vi "LABVIEW ECG.vi"() -> ()   [LabVIEW 2016]
uses:
  <vilib>/Instr/_visa.llb/Select Event Type.ctl
  <vilib>/Instr/_visa.llb/VISA Configure Serial Port (Instr).vi
  <vilib>/express/express analysis/Spectral/Block/exnSpectralBlock spectral measurements peak poly.vi
  <vilib>/express/express analysis/Spectral/Block/exnSpectralBlock spectral measurements peak WFM.vi
  <vilib>/express/express analysis/Spectral/Block/exnSpectralBlock spectral measurements peak DDT.vi
  <vilib>/express/express analysis/Spectral/XNode/ExpressSpectralMeasurementsBlockNode.xnode
  <vilib>/measure/NI_MABase.lvlib
  <vilib>/ptbypt/NI_PtbyPt.lvlib
panel:
  out "?":bool
  in  "?":bool
  in  "Tab Control":T1(tab)
  in  "COM Port":refnum<visa-resource-name>="COM7"
  in  "Parametres VISA":T2={"baud rate (9600)"=500000, "data bits (8)"=8, "parity (0:none)"=enum."None", "stop bits (10: 1 bit)"=10, "flow control (0:none)"=0} {"stop bits (10: 1 bit)" items=["1.0"=10, "1.5"=15, "2.0"=20]; "flow control (0:none)" items=["None", "XON/XOFF", "RTS/CTS", "XON/XOFF & RTS/CTS", "DTR/DSR", "XON/XOFF & DTR/DSR"]}
  out "Signal bruité":waveform(dbl)(graph)={"t0"=timestamp(1563.0 s since 1904-01-01), "dt"=0.001, "Y"=array[1000 elements]}
  out "Signal filtré":dynamicdata(graph)=[{"t0"=timestamp(1563.0 s since 1904-01-01), "dt"=0.001, "Y"=array[1000 elements], "attributes"=variant("NI_ChannelName"=variant(string "Filtered"))}]
  in  "Frequence Reseau":dbl=10.0 format="%0.2p"
  in  "Frequence de coupure":dbl=0.125 format="%0.3f"
  out "Table 2":string[][](table)=[["20/06/2020 23:30:40", "98,000000"], ["20/06/2020 23:30:41", "32,000000"], ["20/06/2020 23:30:41", "32,000000"], ["20/06/2020 23:30:41", "32,000000"], ["20/06/2020 23:30:41", "33,000000"], ["20/06/2020 23:30:41", "33,000000"], ["20/06/2020 23:30:41", "33,000000"], ["20/06/2020 23:30:41", "33,000000"], ["20/06/2020 23:30:41", "33,000000"], ["20/06/2020 23:30:41", "34,000000"], ["20/06/2020 23:30:41", "35,000000"], ["20/06/2020 23:30:41", "35,000000"], ["20/06/2020 23:30:41", "34,000000"], ["20/06/2020 23:30:41", "33,000000"], ["20/06/2020 23:30:41", "35,000000"], ["20/06/2020 23:30:41", "34,000000"], ["20/06/2020 23:30:41", "33,000000"], ["20/06/2020 23:30:41", "34,000000"], ["20/06/2020 23:30:41", "34,000000"], ["20/06/2020 23:30:41", "33,000000"], ["20/06/2020 23:30:41", "33,000000"], ["20/06/2020 23:30:41", "33,000000"], ["20/06/2020 23:30:41", "34,000000"], ["20/06/2020 23:30:41", "34,000000"], ["20/06/2020 23:30:41", "34,000000"], ["20/06/2020 23:30:41", "35,000000"], ["20/06/2020 23:30:41", "35,000000"], ["20/06/2020 23:30:41", "34,000000"], ["20/06/2020 23:30:41", "36,000000"], ["20/06/2020 23:30:41", "35,000000"], ["20/06/2020 23:30:41", "35,000000"], ["20/06/2020 23:30:41", "36,000000"], ["20/06/2020 23:30:41", "36,000000"], ["20/06/2020 23:30:41", "38,000000"], ["20/06/2020 23:30:41", "37,000000"], ["20/06/2020 23:30:41", "38,000000"], ["20/06/2020 23:30:41", "38,000000"], ["20/06/2020 23:30:41", "38,000000"], ["20/06/2020 23:30:41", "40,000000"], ["20/06/2020 23:30:41", "40,000000"], ["20/06/2020 23:30:41", "40,000000"], ["20/06/2020 23:30:41", "41,000000"], ["20/06/2020 23:30:41", "42,000000"], ["20/06/2020 23:30:41", "41,000000"], ["20/06/2020 23:30:41", "41,000000"], ["20/06/2020 23:30:41", "43,000000"], ["20/06/2020 23:30:41", "42,000000"], ["20/06/2020 23:30:41", "43,000000"], ["20/06/2020 23:30:41", "44,000000"], ["20/06/2020 23:30:41", "45,000000"], ["20/06/2020 23:30:41", "45,000000"], ["20/06/2020 23:30:41", "46,000000"], ["20/06/2020 23:30:41", "45,000000"], ["20/06/2020 23:30:41", "47,000000"], ["20/06/2020 23:30:41", "47,000000"], ["20/06/2020 23:30:41", "47,000000"], ["20/06/2020 23:30:41", "47,000000"], ["20/06/2020 23:30:41", "48,000000"], ["20/06/2020 23:30:41", "49,000000"], ["20/06/2020 23:30:41", "49,000000"], ["20/06/2020 23:30:41", "50,000000"], ["20/06/2020 23:30:41", "50,000000"], ["20/06/2020 23:30:41", "49,000000"], ["20/06/2020 23:30:41", "48,000000"], ["20/06/2020 23:30:41", "49,000000"], ["20/06/2020 23:30:41", "48,000000"], ["20/06/2020 23:30:41", "49,000000"], ["20/06/2020 23:30:41", "49,000000"], ["20/06/2020 23:30:41", "50,000000"], ["20/06/2020 23:30:41", "50,000000"], ["20/06/2020 23:30:41", "50,000000"], ["20/06/2020 23:30:41", "50,000000"], ["20/06/2020 23:30:41", "51,000000"], ["20/06/2020 23:30:41", "50,000000"], ["20/06/2020 23:30:41", "50,000000"], ["20/06/2020 23:30:41", "49,000000"], ["20/06/2020 23:30:41", "49,000000"], ["20/06/2020 23:30:41", "48,000000"], ["20/06/2020 23:30:41", "47,000000"], ["20/06/2020 23:30:41", "47,000000"], ["20/06/2020 23:30:41", "46,000000"], ["20/06/2020 23:30:41", "46,000000"], ["20/06/2020 23:30:41", "44,000000"], ["20/06/2020 23:30:41", "42,000000"], ["20/06/2020 23:30:41", "42,000000"], ["20/06/2020 23:30:41", "39,000000"], ["20/06/2020 23:30:41", "39,000000"], ["20/06/2020 23:30:41", "39,000000"], ["20/06/2020 23:30:41", "38,000000"], ["20/06/2020 23:30:41", "39,000000"], ["20/06/2020 23:30:41", "36,000000"], ["20/06/2020 23:30:41", "34,000000"], ["20/06/2020 23:30:41", "34,000000"], ["20/06/2020 23:30:41", "33,000000"], ["20/06/2020 23:30:41", "32,000000"], ["20/06/2020 23:30:42", "31,000000"], ["20/06/2020 23:30:42", "30,000000"], ["20/06/2020 23:30:42", "30,000000"], ["20/06/2020 23:30:42", "31,000000"], ["20/06/2020 23:30:42", "30,000000"], ["20/06/2020 23:30:42", "30,000000"], ["20/06/2020 23:30:42", "29,000000"], ["20/06/2020 23:30:42", "29,000000"], ["20/06/2020 23:30:42", "27,000000"], ["20/06/2020 23:30:42", "27,000000"], ["20/06/2020 23:30:42", "27,000000"], ["20/06/2020 23:30:42", "25,000000"], ["20/06/2020 23:30:42", "25,000000"], ["20/06/2020 23:30:42", "24,000000"], ["20/06/2020 23:30:42", "26,000000"], ["20/06/2020 23:30:42", "25,000000"], ["20/06/2020 23:30:42", "25,000000"], ["20/06/2020 23:30:42", "25,000000"], ["20/06/2020 23:30:42", "24,000000"], ["20/06/2020 23:30:42", "25,000000"], ["20/06/2020 23:30:42", "24,000000"], ["20/06/2020 23:30:42", "24,000000"], ["20/06/2020 23:30:42", "24,000000"], ["20/06/2020 23:30:42", "24,000000"], ["20/06/2020 23:30:42", "25,000000"], ["20/06/2020 23:30:42", "23,000000"], ["20/06/2020 23:30:42", "25,000000"], ["20/06/2020 23:30:42", "24,000000"], ["20/06/2020 23:30:42", "23,000000"], ["20/06/2020 23:30:42", "23,000000"], ["20/06/2020 23:30:42", "22,000000"], ["20/06/2020 23:30:42", "21,000000"], ["20/06/2020 23:30:42", "20,000000"], ["20/06/2020 23:30:42", "22,000000"], ["20/06/2020 23:30:42", "21,000000"], ["20/06/2020 23:30:42", "21,000000"], ["20/06/2020 23:30:42", "21,000000"], ["20/06/2020 23:30:42", "19,000000"], ["20/06/2020 23:30:42", "18,000000"], ["20/06/2020 23:30:42", "19,000000"], ["20/06/2020 23:30:42", "19,000000"], ["20/06/2020 23:30:42", "19,000000"], ["20/06/2020 23:30:42", "19,000000"], ["20/06/2020 23:30:42", "18,000000"], ["20/06/2020 23:30:42", "20,000000"], ["20/06/2020 23:30:42", "19,000000"], ["20/06/2020 23:30:42", "19,000000"], ["20/06/2020 23:30:42", "21,000000"], ["20/06/2020 23:30:42", "20,000000"], ["20/06/2020 23:30:42", "20,000000"], ["20/06/2020 23:30:42", "19,000000"], ["20/06/2020 23:30:42", "19,000000"], ["20/06/2020 23:30:42", "21,000000"], ["20/06/2020 23:30:42", "21,000000"], ["20/06/2020 23:30:42", "20,000000"], ["20/06/2020 23:30:42", "22,000000"], ["20/06/2020 23:30:42", "23,000000"], ["20/06/2020 23:30:42", "22,000000"], ["20/06/2020 23:30:42", "20,000000"], ["20/06/2020 23:30:42", "21,000000"], ["20/06/2020 23:30:42", "21,000000"], ["20/06/2020 23:30:42", "21,000000"], ["20/06/2020 23:30:42", "23,000000"], ["20/06/2020 23:30:42", "23,000000"], ["20/06/2020 23:30:42", "23,000000"], ["20/06/2020 23:30:42", "21,000000"], ["20/06/2020 23:30:42", "21,000000"], ["20/06/2020 23:30:42", "22,000000"], ["20/06/2020 23:30:42", "22,000000"], ["20/06/2020 23:30:42", "22,000000"], ["20/06/2020 23:30:42", "22,000000"], ["20/06/2020 23:30:42", "22,000000"], ["20/06/2020 23:30:42", "22,000000"], ["20/06/2020 23:30:42", "23,000000"], ["20/06/2020 23:30:42", "23,000000"], ["20/06/2020 23:30:42", "22,000000"], ["20/06/2020 23:30:42", "22,000000"], ["20/06/2020 23:30:42", "23,000000"], ["20/06/2020 23:30:42", "22,000000"], ["20/06/2020 23:30:42", "23,000000"], ["20/06/2020 23:30:42", "22,000000"], ["20/06/2020 23:30:42", "22,000000"], ["20/06/2020 23:30:42", "23,000000"], ["20/06/2020 23:30:42", "23,000000"], ["20/06/2020 23:30:42", "21,000000"], ["20/06/2020 23:30:42", "22,000000"], ["20/06/2020 23:30:42", "22,000000"], ["20/06/2020 23:30:42", "23,000000"], ["20/06/2020 23:30:42", "21,000000"], ["20/06/2020 23:30:42", "20,000000"], ["20/06/2020 23:30:42", "22,000000"], ["20/06/2020 23:30:42", "22,000000"], ["20/06/2020 23:30:42", "22,000000"], ["20/06/2020 23:30:42", "23,000000"], ["20/06/2020 23:30:42", "23,000000"], ["20/06/2020 23:30:42", "22,000000"], ["20/06/2020 23:30:42", "22,000000"], ["20/06/2020 23:30:42", "23,000000"], ["20/06/2020 23:30:42", "23,000000"], ["20/06/2020 23:30:42", "23,000000"], ["20/06/2020 23:30:42", "22,000000"], ["20/06/2020 23:30:42", "21,000000"], ["20/06/2020 23:30:42", "21,000000"], ["20/06/2020 23:30:42", "20,000000"], ["20/06/2020 23:30:42", "23,000000"], ["20/06/2020 23:30:42", "21,000000"], ["20/06/2020 23:30:42", "19,000000"], ["20/06/2020 23:30:42", "19,000000"], ["20/06/2020 23:30:42", "18,000000"], ["20/06/2020 23:30:42", "18,000000"], ["20/06/2020 23:30:42", "19,000000"], ["20/06/2020 23:30:42", "19,000000"], ["20/06/2020 23:30:42", "19,000000"], ["20/06/2020 23:30:42", "19,000000"], ["20/06/2020 23:30:42", "19,000000"], ["20/06/2020 23:30:42", "19,000000"], ["20/06/2020 23:30:42", "19,000000"], ["20/06/2020 23:30:42", "19,000000"], ["20/06/2020 23:30:42", "18,000000"], ["20/06/2020 23:30:42", "19,000000"], ["20/06/2020 23:30:42", "18,000000"], ["20/06/2020 23:30:42", "17,000000"], ["20/06/2020 23:30:42", "18,000000"], ["20/06/2020 23:30:42", "18,000000"], ["20/06/2020 23:30:42", "18,000000"], ["20/06/2020 23:30:42", "18,000000"], ["20/06/2020 23:30:42", "19,000000"], ["20/06/2020 23:30:42", "19,000000"], ["20/06/2020 23:30:42", "18,000000"], ["20/06/2020 23:30:42", "19,000000"], ["20/06/2020 23:30:42", "18,000000"], ["20/06/2020 23:30:42", "19,000000"], ["20/06/2020 23:30:42", "18,000000"], ["20/06/2020 23:30:42", "18,000000"], ["20/06/2020 23:30:42", "18,000000"], ["20/06/2020 23:30:42", "18,000000"], ["20/06/2020 23:30:42", "18,000000"], ["20/06/2020 23:30:42", "17,000000"], ["20/06/2020 23:30:42", "16,000000"], ["20/06/2020 23:30:42", "17,000000"], ["20/06/2020 23:30:42", "17,000000"], ["20/06/2020 23:30:42", "16,000000"], ["20/06/2020 23:30:42", "17,000000"], ["20/06/2020 23:30:42", "18,000000"], ["20/06/2020 23:30:42", "18,000000"], ["20/06/2020 23:30:42", "18,000000"], ["20/06/2020 23:30:42", "17,000000"], ["20/06/2020 23:30:42", "17,000000"], ["20/06/2020 23:30:42", "17,000000"], ["20/06/2020 23:30:42", "17,000000"], ["20/06/2020 23:30:42", "17,000000"], ["20/06/2020 23:30:42", "18,000000"], ["20/06/2020 23:30:42", "17,000000"], ["20/06/2020 23:30:42", "16,000000"], ["20/06/2020 23:30:42", "16,000000"], ["20/06/2020 23:30:42", "16,000000"], ["20/06/2020 23:30:42", "17,000000"], ["20/06/2020 23:30:42", "18,000000"], ["20/06/2020 23:30:42", "17,000000"], ["20/06/2020 23:30:42", "17,000000"], ["20/06/2020 23:30:42", "17,000000"], ["20/06/2020 23:30:42", "17,000000"], ["20/06/2020 23:30:42", "16,000000"], ["20/06/2020 23:30:42", "17,000000"], ["20/06/2020 23:30:42", "17,000000"], ["20/06/2020 23:30:42", "17,000000"], ["20/06/2020 23:30:42", "18,000000"], ["20/06/2020 23:30:42", "17,000000"], ["20/06/2020 23:30:42", "16,000000"], ["20/06/2020 23:30:42", "16,000000"], ["20/06/2020 23:30:42", "16,000000"], ["20/06/2020 23:30:42", "17,000000"], ["20/06/2020 23:30:42", "18,000000"], ["20/06/2020 23:30:42", "17,000000"], ["20/06/2020 23:30:42", "16,000000"], ["20/06/2020 23:30:42", "17,000000"], ["20/06/2020 23:30:42", "17,000000"], ["20/06/2020 23:30:42", "17,000000"], ["20/06/2020 23:30:42", "17,000000"], ["20/06/2020 23:30:42", "15,000000"], ["20/06/2020 23:30:42", "16,000000"], ["20/06/2020 23:30:42", "16,000000"], ["20/06/2020 23:30:42", "16,000000"], ["20/06/2020 23:30:42", "17,000000"], ["20/06/2020 23:30:42", "16,000000"], ["20/06/2020 23:30:42", "16,000000"], ["20/06/2020 23:30:42", "16,000000"], ["20/06/2020 23:30:42", "16,000000"], ["20/06/2020 23:30:42", "16,000000"], ["20/06/2020 23:30:42", "15,000000"], ["20/06/2020 23:30:42", "16,000000"], ["20/06/2020 23:30:42", "16,000000"], ["20/06/2020 23:30:42", "16,000000"], ["20/06/2020 23:30:42", "16,000000"], ["20/06/2020 23:30:42", "16,000000"], ["20/06/2020 23:30:42", "17,000000"], ["20/06/2020 23:30:42", "16,000000"], ["20/06/2020 23:30:42", "17,000000"], ["20/06/2020 23:30:42", "17,000000"], ["20/06/2020 23:30:42", "17,000000"], ["20/06/2020 23:30:42", "17,000000"], ["20/06/2020 23:30:42", "16,000000"], ["20/06/2020 23:30:42", "16,000000"], ["20/06/2020 23:30:42", "16,000000"], ["20/06/2020 23:30:42", "16,000000"], ["20/06/2020 23:30:42", "17,000000"], ["20/06/2020 23:30:42", "16,000000"], ["20/06/2020 23:30:42", "17,000000"], ["20/06/2020 23:30:42", "16,000000"], ["20/06/2020 23:30:42", "16,000000"], ["20/06/2020 23:30:42", "16,000000"], ["20/06/2020 23:30:42", "16,000000"], ["20/06/2020 23:30:42", "16,000000"], ["20/06/2020 23:30:42", "17,000000"], ["20/06/2020 23:30:42", "17,000000"], ["20/06/2020 23:30:42", "16,000000"], ["20/06/2020 23:30:42", "16,000000"], ["20/06/2020 23:30:42", "16,000000"], ["20/06/2020 23:30:42", "14,000000"], ["20/06/2020 23:30:42", "15,000000"], ["20/06/2020 23:30:42", "15,000000"], ["20/06/2020 23:30:42", "16,000000"], ["20/06/2020 23:30:42", "16,000000"], ["20/06/2020 23:30:42", "18,000000"], ["20/06/2020 23:30:42", "19,000000"], ["20/06/2020 23:30:42", "17,000000"], ["20/06/2020 23:30:42", "18,000000"], ["20/06/2020 23:30:42", "17,000000"], ["20/06/2020 23:30:42", "16,000000"], ["20/06/2020 23:30:42", "16,000000"], ["20/06/2020 23:30:42", "17,000000"], ["20/06/2020 23:30:42", "17,000000"], ["20/06/2020 23:30:42", "18,000000"], ["20/06/2020 23:30:42", "19,000000"], ["20/06/2020 23:30:42", "20,000000"], ["20/06/2020 23:30:42", "21,000000"], ["20/06/2020 23:30:42", "22,000000"], ["20/06/2020 23:30:42", "23,000000"], ["20/06/2020 23:30:42", "22,000000"], ["20/06/2020 23:30:42", "22,000000"], ["20/06/2020 23:30:42", "24,000000"], ["20/06/2020 23:30:42", "25,000000"], ["20/06/2020 23:30:42", "26,000000"], ["20/06/2020 23:30:42", "26,000000"], ["20/06/2020 23:30:42", "27,000000"], ["20/06/2020 23:30:42", "27,000000"], ["20/06/2020 23:30:42", "29,000000"], ["20/06/2020 23:30:42", "29,000000"], ["20/06/2020 23:30:42", "27,000000"], ["20/06/2020 23:30:42", "27,000000"], ["20/06/2020 23:30:42", "26,000000"], ["20/06/2020 23:30:42", "25,000000"], ["20/06/2020 23:30:42", "23,000000"], ["20/06/2020 23:30:42", "24,000000"], ["20/06/2020 23:30:42", "23,000000"], ["20/06/2020 23:30:42", "23,000000"], ["20/06/2020 23:30:42", "22,000000"], ["20/06/2020 23:30:42", "19,000000"], ["20/06/2020 23:30:42", "19,000000"], ["20/06/2020 23:30:42", "18,000000"], ["20/06/2020 23:30:42", "16,000000"], ["20/06/2020 23:30:42", "15,000000"], ["20/06/2020 23:30:42", "14,000000"], ["20/06/2020 23:30:42", "16,000000"], ["20/06/2020 23:30:42", "15,000000"], ["20/06/2020 23:30:42", "14,000000"], ["20/06/2020 23:30:42", "14,000000"], ["20/06/2020 23:30:42", "14,000000"], ["20/06/2020 23:30:42", "14,000000"], ["20/06/2020 23:30:42", "14,000000"], ["20/06/2020 23:30:42", "15,000000"], ["20/06/2020 23:30:42", "14,000000"], ["20/06/2020 23:30:42", "14,000000"], ["20/06/2020 23:30:42", "13,000000"], ["20/06/2020 23:30:42", "13,000000"], ["20/06/2020 23:30:42", "13,000000"], ["20/06/2020 23:30:42", "14,000000"], ["20/06/2020 23:30:42", "13,000000"], ["20/06/2020 23:30:42", "12,000000"], ["20/06/2020 23:30:42", "13,000000"], ["20/06/2020 23:30:42", "12,000000"], ["20/06/2020 23:30:42", "12,000000"], ["20/06/2020 23:30:42", "11,000000"], ["20/06/2020 23:30:42", "11,000000"], ["20/06/2020 23:30:42", "12,000000"], ["20/06/2020 23:30:42", "13,000000"], ["20/06/2020 23:30:42", "15,000000"], ["20/06/2020 23:30:42", "16,000000"], ["20/06/2020 23:30:42", "16,000000"], ["20/06/2020 23:30:42", "14,000000"], ["20/06/2020 23:30:42", "15,000000"], ["20/06/2020 23:30:42", "20,000000"], ["20/06/2020 23:30:42", "27,000000"], ["20/06/2020 23:30:42", "35,000000"], ["20/06/2020 23:30:42", "45,000000"], ["20/06/2020 23:30:42", "61,000000"], ["20/06/2020 23:30:42", "74,000000"], ["20/06/2020 23:30:42", "82,000000"], ["20/06/2020 23:30:42", "96,000000"], ["20/06/2020 23:30:42", "110,000000"], ["20/06/2020 23:30:42", "122,000000"], ["20/06/2020 23:30:42", "132,000000"], ["20/06/2020 23:30:42", "139,000000"], ["20/06/2020 23:30:42", "140,000000"], ["20/06/2020 23:30:42", "130,000000"], ["20/06/2020 23:30:42", "116,000000"], ["20/06/2020 23:30:42", "99,000000"], ["20/06/2020 23:30:42", "78,000000"], ["20/06/2020 23:30:42", "56,000000"], ["20/06/2020 23:30:42", "39,000000"], ["20/06/2020 23:30:42", "24,000000"], ["20/06/2020 23:30:42", "23,000000"], ["20/06/2020 23:30:42", "21,000000"], ["20/06/2020 23:30:42", "18,000000"], ["20/06/2020 23:30:42", "17,000000"], ["20/06/2020 23:30:42", "14,000000"], ["20/06/2020 23:30:42", "14,000000"], ["20/06/2020 23:30:42", "12,000000"], ["20/06/2020 23:30:42", "11,000000"], ["20/06/2020 23:30:42", "11,000000"], ["20/06/2020 23:30:42", "11,000000"], ["20/06/2020 23:30:42", "11,000000"], ["20/06/2020 23:30:42", "11,000000"], ["20/06/2020 23:30:42", "13,000000"], ["20/06/2020 23:30:42", "15,000000"], ["20/06/2020 23:30:42", "16,000000"], ["20/06/2020 23:30:42", "16,000000"], ["20/06/2020 23:30:42", "16,000000"], ["20/06/2020 23:30:42", "16,000000"], ["20/06/2020 23:30:42", "16,000000"], ["20/06/2020 23:30:42", "15,000000"], ["20/06/2020 23:30:42", "15,000000"], ["20/06/2020 23:30:42", "15,000000"], ["20/06/2020 23:30:42", "16,000000"], ["20/06/2020 23:30:42", "16,000000"], ["20/06/2020 23:30:42", "15,000000"], ["20/06/2020 23:30:42", "16,000000"], ["20/06/2020 23:30:42", "16,000000"], ["20/06/2020 23:30:42", "16,000000"], ["20/06/2020 23:30:42", "16,000000"], ["20/06/2020 23:30:42", "15,000000"], ["20/06/2020 23:30:42", "16,000000"], ["20/06/2020 23:30:42", "17,000000"], ["20/06/2020 23:30:42", "17,000000"], ["20/06/2020 23:30:42", "17,000000"], ["20/06/2020 23:30:42", "16,000000"], ["20/06/2020 23:30:42", "17,000000"], ["20/06/2020 23:30:42", "18,000000"], ["20/06/2020 23:30:42", "17,000000"], ["20/06/2020 23:30:42", "16,000000"], ["20/06/2020 23:30:42", "17,000000"], ["20/06/2020 23:30:42", "17,000000"], ["20/06/2020 23:30:42", "16,000000"], ["20/06/2020 23:30:42", "17,000000"], ["20/06/2020 23:30:42", "17,000000"], ["20/06/2020 23:30:42", "17,000000"], ["20/06/2020 23:30:42", "17,000000"], ["20/06/2020 23:30:42", "18,000000"], ["20/06/2020 23:30:42", "17,000000"], ["20/06/2020 23:30:42", "17,000000"], ["20/06/2020 23:30:43", "16,000000"], ["20/06/2020 23:30:43", "16,000000"], ["20/06/2020 23:30:43", "16,000000"], ["20/06/2020 23:30:43", "16,000000"], ["20/06/2020 23:30:43", "16,000000"], ["20/06/2020 23:30:43", "17,000000"], ["20/06/2020 23:30:43", "18,000000"], ["20/06/2020 23:30:43", "18,000000"], ["20/06/2020 23:30:43", "17,000000"], ["20/06/2020 23:30:43", "18,000000"], ["20/06/2020 23:30:43", "18,000000"], ["20/06/2020 23:30:43", "17,000000"], ["20/06/2020 23:30:43", "17,000000"], ["20/06/2020 23:30:43", "18,000000"], ["20/06/2020 23:30:43", "18,000000"], ["20/06/2020 23:30:43", "18,000000"], ["20/06/2020 23:30:43", "18,000000"], ["20/06/2020 23:30:43", "18,000000"], ["20/06/2020 23:30:43", "17,000000"], ["20/06/2020 23:30:43", "18,000000"], ["20/06/2020 23:30:43", "17,000000"], ["20/06/2020 23:30:43", "18,000000"], ["20/06/2020 23:30:43", "19,000000"], ["20/06/2020 23:30:43", "19,000000"], ["20/06/2020 23:30:43", "19,000000"], ["20/06/2020 23:30:43", "20,000000"], ["20/06/2020 23:30:43", "20,000000"], ["20/06/2020 23:30:43", "19,000000"], ["20/06/2020 23:30:43", "19,000000"], ["20/06/2020 23:30:43", "21,000000"], ["20/06/2020 23:30:43", "22,000000"], ["20/06/2020 23:30:43", "21,000000"], ["20/06/2020 23:30:43", "22,000000"], ["20/06/2020 23:30:43", "22,000000"], ["20/06/2020 23:30:43", "22,000000"], ["20/06/2020 23:30:43", "22,000000"], ["20/06/2020 23:30:43", "21,000000"], ["20/06/2020 23:30:43", "21,000000"], ["20/06/2020 23:30:43", "21,000000"], ["20/06/2020 23:30:43", "22,000000"], ["20/06/2020 23:30:43", "23,000000"], ["20/06/2020 23:30:43", "23,000000"], ["20/06/2020 23:30:43", "23,000000"], ["20/06/2020 23:30:43", "25,000000"], ["20/06/2020 23:30:43", "25,000000"], ["20/06/2020 23:30:43", "26,000000"], ["20/06/2020 23:30:43", "27,000000"], ["20/06/2020 23:30:43", "26,000000"], ["20/06/2020 23:30:43", "26,000000"], ["20/06/2020 23:30:43", "26,000000"], ["20/06/2020 23:30:43", "27,000000"], ["20/06/2020 23:30:43", "27,000000"], ["20/06/2020 23:30:43", "28,000000"], ["20/06/2020 23:30:43", "29,000000"], ["20/06/2020 23:30:43", "29,000000"], ["20/06/2020 23:30:43", "30,000000"], ["20/06/2020 23:30:43", "30,000000"], ["20/06/2020 23:30:43", "31,000000"], ["20/06/2020 23:30:43", "31,000000"], ["20/06/2020 23:30:43", "32,000000"], ["20/06/2020 23:30:43", "32,000000"], ["20/06/2020 23:30:43", "33,000000"], ["20/06/2020 23:30:43", "33,000000"], ["20/06/2020 23:30:43", "35,000000"], ["20/06/2020 23:30:43", "36,000000"], ["20/06/2020 23:30:43", "35,000000"], ["20/06/2020 23:30:43", "37,000000"], ["20/06/2020 23:30:43", "38,000000"], ["20/06/2020 23:30:43", "37,000000"], ["20/06/2020 23:30:43", "37,000000"], ["20/06/2020 23:30:43", "37,000000"], ["20/06/2020 23:30:43", "37,000000"], ["20/06/2020 23:30:43", "37,000000"], ["20/06/2020 23:30:43", "38,000000"], ["20/06/2020 23:30:43", "37,000000"], ["20/06/2020 23:30:43", "37,000000"], ["20/06/2020 23:30:43", "38,000000"], ["20/06/2020 23:30:43", "39,000000"], ["20/06/2020 23:30:43", "38,000000"], ["20/06/2020 23:30:43", "37,000000"], ["20/06/2020 23:30:43", "38,000000"], ["20/06/2020 23:30:43", "37,000000"], ["20/06/2020 23:30:43", "35,000000"], ["20/06/2020 23:30:43", "36,000000"], ["20/06/2020 23:30:43", "35,000000"], ["20/06/2020 23:30:43", "35,000000"], ["20/06/2020 23:30:43", "35,000000"], ["20/06/2020 23:30:43", "35,000000"], ["20/06/2020 23:30:43", "34,000000"], ["20/06/2020 23:30:43", "33,000000"], ["20/06/2020 23:30:43", "31,000000"], ["20/06/2020 23:30:43", "31,000000"], ["20/06/2020 23:30:43", "31,000000"], ["20/06/2020 23:30:43", "30,000000"], ["20/06/2020 23:30:43", "29,000000"], ["20/06/2020 23:30:43", "28,000000"], ["20/06/2020 23:30:43", "27,000000"], ["20/06/2020 23:30:43", "27,000000"], ["20/06/2020 23:30:43", "26,000000"], ["20/06/2020 23:30:43", "26,000000"], ["20/06/2020 23:30:43", "23,000000"], ["20/06/2020 23:30:43", "23,000000"], ["20/06/2020 23:30:43", "22,000000"], ["20/06/2020 23:30:43", "22,000000"], ["20/06/2020 23:30:43", "21,000000"], ["20/06/2020 23:30:43", "21,000000"], ["20/06/2020 23:30:43", "21,000000"], ["20/06/2020 23:30:43", "19,000000"], ["20/06/2020 23:30:43", "19,000000"], ["20/06/2020 23:30:43", "19,000000"], ["20/06/2020 23:30:43", "17,000000"], ["20/06/2020 23:30:43", "17,000000"], ["20/06/2020 23:30:43", "16,000000"], ["20/06/2020 23:30:43", "17,000000"], ["20/06/2020 23:30:43", "17,000000"], ["20/06/2020 23:30:43", "17,000000"], ["20/06/2020 23:30:43", "18,000000"], ["20/06/2020 23:30:43", "18,000000"], ["20/06/2020 23:30:43", "17,000000"], ["20/06/2020 23:30:43", "17,000000"], ["20/06/2020 23:30:43", "18,000000"], ["20/06/2020 23:30:43", "18,000000"], ["20/06/2020 23:30:43", "17,000000"], ["20/06/2020 23:30:43", "19,000000"], ["20/06/2020 23:30:43", "19,000000"], ["20/06/2020 23:30:43", "18,000000"], ["20/06/2020 23:30:43", "16,000000"], ["20/06/2020 23:30:43", "17,000000"], ["20/06/2020 23:30:43", "17,000000"], ["20/06/2020 23:30:43", "17,000000"], ["20/06/2020 23:30:43", "17,000000"], ["20/06/2020 23:30:43", "17,000000"], ["20/06/2020 23:30:43", "16,000000"], ["20/06/2020 23:30:43", "16,000000"], ["20/06/2020 23:30:43", "16,000000"], ["20/06/2020 23:30:43", "17,000000"], ["20/06/2020 23:30:43", "17,000000"], ["20/06/2020 23:30:43", "16,000000"], ["20/06/2020 23:30:43", "16,000000"], ["20/06/2020 23:30:43", "16,000000"], ["20/06/2020 23:30:43", "16,000000"], ["20/06/2020 23:30:43", "15,000000"], ["20/06/2020 23:30:43", "15,000000"], ["20/06/2020 23:30:43", "15,000000"], ["20/06/2020 23:30:43", "16,000000"], ["20/06/2020 23:30:43", "15,000000"], ["20/06/2020 23:30:43", "17,000000"], ["20/06/2020 23:30:43", "16,000000"], ["20/06/2020 23:30:43", "14,000000"], ["20/06/2020 23:30:43", "14,000000"], ["20/06/2020 23:30:43", "14,000000"], ["20/06/2020 23:30:43", "14,000000"], ["20/06/2020 23:30:43", "14,000000"], ["20/06/2020 23:30:43", "14,000000"], ["20/06/2020 23:30:43", "14,000000"], ["20/06/2020 23:30:43", "14,000000"], ["20/06/2020 23:30:43", "14,000000"], ["20/06/2020 23:30:43", "15,000000"], ["20/06/2020 23:30:43", "14,000000"], ["20/06/2020 23:30:43", "14,000000"], ["20/06/2020 23:30:43", "14,000000"], ["20/06/2020 23:30:43", "15,000000"], ["20/06/2020 23:30:43", "15,000000"], ["20/06/2020 23:30:43", "16,000000"], ["20/06/2020 23:30:43", "15,000000"], ["20/06/2020 23:30:43", "16,000000"], ["20/06/2020 23:30:43", "16,000000"], ["20/06/2020 23:30:43", "15,000000"], ["20/06/2020 23:30:43", "15,000000"], ["20/06/2020 23:30:43", "15,000000"], ["20/06/2020 23:30:43", "15,000000"], ["20/06/2020 23:30:43", "15,000000"], ["20/06/2020 23:30:43", "15,000000"], ["20/06/2020 23:30:43", "16,000000"], ["20/06/2020 23:30:43", "15,000000"], ["20/06/2020 23:30:43", "16,000000"], ["20/06/2020 23:30:43", "16,000000"], ["20/06/2020 23:30:43", "16,000000"], ["20/06/2020 23:30:43", "16,000000"], ["20/06/2020 23:30:43", "16,000000"], ["20/06/2020 23:30:43", "17,000000"], ["20/06/2020 23:30:43", "16,000000"], ["20/06/2020 23:30:43", "15,000000"], ["20/06/2020 23:30:43", "15,000000"], ["20/06/2020 23:30:43", "15,000000"], ["20/06/2020 23:30:43", "14,000000"], ["20/06/2020 23:30:43", "15,000000"], ["20/06/2020 23:30:43", "16,000000"], ["20/06/2020 23:30:43", "16,000000"], ["20/06/2020 23:30:43", "14,000000"], ["20/06/2020 23:30:43", "15,000000"], ["20/06/2020 23:30:43", "14,000000"], ["20/06/2020 23:30:43", "14,000000"], ["20/06/2020 23:30:43", "15,000000"], ["20/06/2020 23:30:43", "15,000000"], ["20/06/2020 23:30:43", "16,000000"], ["20/06/2020 23:30:43", "16,000000"], ["20/06/2020 23:30:43", "17,000000"], ["20/06/2020 23:30:43", "16,000000"], ["20/06/2020 23:30:43", "15,000000"], ["20/06/2020 23:30:43", "15,000000"], ["20/06/2020 23:30:43", "15,000000"], ["20/06/2020 23:30:43", "16,000000"], ["20/06/2020 23:30:43", "16,000000"], ["20/06/2020 23:30:43", "16,000000"], ["20/06/2020 23:30:43", "15,000000"], ["20/06/2020 23:30:43", "16,000000"], ["20/06/2020 23:30:43", "15,000000"], ["20/06/2020 23:30:43", "16,000000"], ["20/06/2020 23:30:43", "16,000000"], ["20/06/2020 23:30:43", "15,000000"], ["20/06/2020 23:30:43", "15,000000"], ["20/06/2020 23:30:43", "15,000000"], ["20/06/2020 23:30:43", "15,000000"], ["20/06/2020 23:30:43", "15,000000"], ["20/06/2020 23:30:43", "16,000000"], ["20/06/2020 23:30:43", "16,000000"], ["20/06/2020 23:30:43", "16,000000"], ["20/06/2020 23:30:43", "16,000000"], ["20/06/2020 23:30:43", "16,000000"], ["20/06/2020 23:30:43", "16,000000"], ["20/06/2020 23:30:43", "16,000000"], ["20/06/2020 23:30:43", "16,000000"], ["20/06/2020 23:30:43", "15,000000"], ["20/06/2020 23:30:43", "14,000000"], ["20/06/2020 23:30:43", "13,000000"], ["20/06/2020 23:30:43", "14,000000"], ["20/06/2020 23:30:43", "13,000000"], ["20/06/2020 23:30:43", "13,000000"], ["20/06/2020 23:30:43", "13,000000"], ["20/06/2020 23:30:43", "14,000000"], ["20/06/2020 23:30:43", "14,000000"], ["20/06/2020 23:30:43", "15,000000"], ["20/06/2020 23:30:43", "14,000000"], ["20/06/2020 23:30:43", "15,000000"], ["20/06/2020 23:30:43", "15,000000"], ["20/06/2020 23:30:43", "15,000000"], ["20/06/2020 23:30:43", "14,000000"], ["20/06/2020 23:30:43", "15,000000"], ["20/06/2020 23:30:43", "15,000000"], ["20/06/2020 23:30:43", "15,000000"], ["20/06/2020 23:30:43", "14,000000"], ["20/06/2020 23:30:43", "14,000000"], ["20/06/2020 23:30:43", "16,000000"], ["20/06/2020 23:30:43", "14,000000"], ["20/06/2020 23:30:43", "13,000000"], ["20/06/2020 23:30:43", "12,000000"], ["20/06/2020 23:30:43", "13,000000"], ["20/06/2020 23:30:43", "13,000000"], ["20/06/2020 23:30:43", "13,000000"], ["20/06/2020 23:30:43", "14,000000"], ["20/06/2020 23:30:43", "13,000000"], ["20/06/2020 23:30:43", "13,000000"], ["20/06/2020 23:30:43", "14,000000"], ["20/06/2020 23:30:43", "14,000000"], ["20/06/2020 23:30:43", "14,000000"], ["20/06/2020 23:30:43", "14,000000"], ["20/06/2020 23:30:43", "14,000000"], ["20/06/2020 23:30:43", "14,000000"], ["20/06/2020 23:30:43", "14,000000"], ["20/06/2020 23:30:43", "14,000000"], ["20/06/2020 23:30:43", "13,000000"], ["20/06/2020 23:30:43", "13,000000"], ["20/06/2020 23:30:43", "15,000000"], ["20/06/2020 23:30:43", "15,000000"], ["20/06/2020 23:30:43", "14,000000"], ["20/06/2020 23:30:43", "15,000000"], ["20/06/2020 23:30:43", "15,000000"], ["20/06/2020 23:30:43", "15,000000"], ["20/06/2020 23:30:43", "14,000000"], ["20/06/2020 23:30:43", "15,000000"], ["20/06/2020 23:30:43", "14,000000"], ["20/06/2020 23:30:43", "14,000000"], ["20/06/2020 23:30:43", "15,000000"], ["20/06/2020 23:30:43", "14,000000"], ["20/06/2020 23:30:43", "14,000000"], ["20/06/2020 23:30:43", "14,000000"], ["20/06/2020 23:30:43", "14,000000"], ["20/06/2020 23:30:43", "14,000000"], ["20/06/2020 23:30:43", "14,000000"], ["20/06/2020 23:30:43", "14,000000"], ["20/06/2020 23:30:43", "13,000000"], ["20/06/2020 23:30:43", "13,000000"], ["20/06/2020 23:30:43", "14,000000"], ["20/06/2020 23:30:43", "13,000000"], ["20/06/2020 23:30:43", "12,000000"], ["20/06/2020 23:30:43", "12,000000"], ["20/06/2020 23:30:43", "11,000000"], ["20/06/2020 23:30:43", "11,000000"], ["20/06/2020 23:30:43", "11,000000"], ["20/06/2020 23:30:43", "11,000000"], ["20/06/2020 23:30:43", "10,000000"], ["20/06/2020 23:30:43", "11,000000"], ["20/06/2020 23:30:43", "11,000000"], ["20/06/2020 23:30:43", "12,000000"], ["20/06/2020 23:30:43", "12,000000"], ["20/06/2020 23:30:43", "12,000000"], ["20/06/2020 23:30:43", "13,000000"], ["20/06/2020 23:30:43", "12,000000"], ["20/06/2020 23:30:43", "12,000000"], ["20/06/2020 23:30:43", "12,000000"], ["20/06/2020 23:30:43", "12,000000"], ["20/06/2020 23:30:43", "13,000000"], ["20/06/2020 23:30:43", "14,000000"], ["20/06/2020 23:30:43", "14,000000"], ["20/06/2020 23:30:43", "14,000000"], ["20/06/2020 23:30:43", "16,000000"], ["20/06/2020 23:30:43", "16,000000"], ["20/06/2020 23:30:43", "16,000000"], ["20/06/2020 23:30:43", "17,000000"], ["20/06/2020 23:30:43", "15,000000"], ["20/06/2020 23:30:43", "14,000000"], ["20/06/2020 23:30:43", "14,000000"], ["20/06/2020 23:30:43", "14,000000"], ["20/06/2020 23:30:43", "13,000000"], ["20/06/2020 23:30:43", "14,000000"], ["20/06/2020 23:30:43", "15,000000"], ["20/06/2020 23:30:43", "16,000000"], ["20/06/2020 23:30:43", "15,000000"], ["20/06/2020 23:30:43", "15,000000"], ["20/06/2020 23:30:43", "16,000000"], ["20/06/2020 23:30:43", "16,000000"], ["20/06/2020 23:30:43", "16,000000"], ["20/06/2020 23:30:43", "16,000000"], ["20/06/2020 23:30:43", "15,000000"], ["20/06/2020 23:30:43", "15,000000"], ["20/06/2020 23:30:43", "16,000000"], ["20/06/2020 23:30:43", "17,000000"], ["20/06/2020 23:30:43", "18,000000"], ["20/06/2020 23:30:43", "19,000000"], ["20/06/2020 23:30:43", "20,000000"], ["20/06/2020 23:30:43", "20,000000"], ["20/06/2020 23:30:43", "20,000000"], ["20/06/2020 23:30:43", "21,000000"], ["20/06/2020 23:30:43", "21,000000"], ["20/06/2020 23:30:43", "22,000000"], ["20/06/2020 23:30:43", "24,000000"], ["20/06/2020 23:30:43", "25,000000"], ["20/06/2020 23:30:43", "26,000000"], ["20/06/2020 23:30:43", "26,000000"], ["20/06/2020 23:30:43", "27,000000"], ["20/06/2020 23:30:43", "26,000000"], ["20/06/2020 23:30:43", "27,000000"], ["20/06/2020 23:30:43", "26,000000"], ["20/06/2020 23:30:43", "26,000000"], ["20/06/2020 23:30:43", "25,000000"], ["20/06/2020 23:30:43", "25,000000"], ["20/06/2020 23:30:43", "24,000000"], ["20/06/2020 23:30:43", "23,000000"], ["20/06/2020 23:30:43", "21,000000"], ["20/06/2020 23:30:43", "19,000000"], ["20/06/2020 23:30:43", "18,000000"], ["20/06/2020 23:30:43", "17,000000"], ["20/06/2020 23:30:43", "17,000000"], ["20/06/2020 23:30:43", "16,000000"], ["20/06/2020 23:30:43", "15,000000"], ["20/06/2020 23:30:43", "15,000000"], ["20/06/2020 23:30:43", "14,000000"], ["20/06/2020 23:30:43", "13,000000"], ["20/06/2020 23:30:43", "13,000000"], ["20/06/2020 23:30:44", "12,000000"], ["20/06/2020 23:30:44", "12,000000"], ["20/06/2020 23:30:44", "11,000000"], ["20/06/2020 23:30:44", "12,000000"], ["20/06/2020 23:30:44", "12,000000"], ["20/06/2020 23:30:44", "12,000000"], ["20/06/2020 23:30:44", "11,000000"], ["20/06/2020 23:30:44", "10,000000"], ["20/06/2020 23:30:44", "10,000000"], ["20/06/2020 23:30:44", "9,000000"], ["20/06/2020 23:30:44", "9,000000"], ["20/06/2020 23:30:44", "9,000000"], ["20/06/2020 23:30:44", "9,000000"], ["20/06/2020 23:30:44", "9,000000"], ["20/06/2020 23:30:44", "10,000000"], ["20/06/2020 23:30:44", "10,000000"], ["20/06/2020 23:30:44", "10,000000"], ["20/06/2020 23:30:44", "11,000000"], ["20/06/2020 23:30:44", "10,000000"], ["20/06/2020 23:30:44", "10,000000"], ["20/06/2020 23:30:44", "11,000000"], ["20/06/2020 23:30:44", "13,000000"], ["20/06/2020 23:30:44", "15,000000"], ["20/06/2020 23:30:44", "15,000000"], ["20/06/2020 23:30:44", "13,000000"], ["20/06/2020 23:30:44", "13,000000"], ["20/06/2020 23:30:44", "18,000000"], ["20/06/2020 23:30:44", "25,000000"], ["20/06/2020 23:30:44", "32,000000"], ["20/06/2020 23:30:44", "40,000000"], ["20/06/2020 23:30:44", "56,000000"], ["20/06/2020 23:30:44", "72,000000"], ["20/06/2020 23:30:44", "81,000000"], ["20/06/2020 23:30:44", "96,000000"], ["20/06/2020 23:30:44", "114,000000"], ["20/06/2020 23:30:44", "125,000000"], ["20/06/2020 23:30:44", "135,000000"], ["20/06/2020 23:30:44", "143,000000"], ["20/06/2020 23:30:44", "142,000000"], ["20/06/2020 23:30:44", "132,000000"], ["20/06/2020 23:30:44", "117,000000"], ["20/06/2020 23:30:44", "96,000000"], ["20/06/2020 23:30:44", "73,000000"], ["20/06/2020 23:30:44", "54,000000"], ["20/06/2020 23:30:44", "34,000000"], ["20/06/2020 23:30:44", "19,000000"], ["20/06/2020 23:30:44", "16,000000"], ["20/06/2020 23:30:44", "15,000000"], ["20/06/2020 23:30:44", "11,000000"], ["20/06/2020 23:30:44", "10,000000"], ["20/06/2020 23:30:44", "7,000000"], ["20/06/2020 23:30:44", "6,000000"], ["20/06/2020 23:30:44", "6,000000"], ["20/06/2020 23:30:44", "6,000000"], ["20/06/2020 23:30:44", "9,000000"], ["20/06/2020 23:30:44", "8,000000"], ["20/06/2020 23:30:44", "9,000000"], ["20/06/2020 23:30:44", "10,000000"], ["20/06/2020 23:30:44", "9,000000"], ["20/06/2020 23:30:44", "12,000000"], ["20/06/2020 23:30:44", "11,000000"], ["20/06/2020 23:30:44", "11,000000"], ["20/06/2020 23:30:44", "11,000000"], ["20/06/2020 23:30:44", "11,000000"], ["20/06/2020 23:30:44", "10,000000"], ["20/06/2020 23:30:44", "11,000000"], ["20/06/2020 23:30:44", "11,000000"], ["20/06/2020 23:30:44", "12,000000"], ["20/06/2020 23:30:44", "11,000000"], ["20/06/2020 23:30:44", "11,000000"], ["20/06/2020 23:30:44", "11,000000"], ["20/06/2020 23:30:44", "11,000000"], ["20/06/2020 23:30:44", "11,000000"], ["20/06/2020 23:30:44", "11,000000"], ["20/06/2020 23:30:44", "11,000000"], ["20/06/2020 23:30:44", "11,000000"], ["20/06/2020 23:30:44", "12,000000"], ["20/06/2020 23:30:44", "12,000000"], ["20/06/2020 23:30:44", "11,000000"], ["20/06/2020 23:30:44", "12,000000"], ["20/06/2020 23:30:44", "11,000000"], ["20/06/2020 23:30:44", "11,000000"], ["20/06/2020 23:30:44", "12,000000"], ["20/06/2020 23:30:44", "12,000000"], ["20/06/2020 23:30:44", "11,000000"], ["20/06/2020 23:30:44", "11,000000"], ["20/06/2020 23:30:44", "11,000000"], ["20/06/2020 23:30:44", "11,000000"], ["20/06/2020 23:30:44", "11,000000"], ["20/06/2020 23:30:44", "11,000000"], ["20/06/2020 23:30:44", "12,000000"], ["20/06/2020 23:30:44", "12,000000"], ["20/06/2020 23:30:44", "11,000000"], ["20/06/2020 23:30:44", "12,000000"], ["20/06/2020 23:30:44", "12,000000"], ["20/06/2020 23:30:44", "12,000000"], ["20/06/2020 23:30:44", "12,000000"], ["20/06/2020 23:30:44", "13,000000"], ["20/06/2020 23:30:44", "12,000000"], ["20/06/2020 23:30:44", "14,000000"], ["20/06/2020 23:30:44", "14,000000"], ["20/06/2020 23:30:44", "14,000000"], ["20/06/2020 23:30:44", "13,000000"], ["20/06/2020 23:30:44", "11,000000"], ["20/06/2020 23:30:44", "12,000000"], ["20/06/2020 23:30:44", "13,000000"], ["20/06/2020 23:30:44", "14,000000"], ["20/06/2020 23:30:44", "14,000000"], ["20/06/2020 23:30:44", "13,000000"], ["20/06/2020 23:30:44", "14,000000"], ["20/06/2020 23:30:44", "14,000000"], ["20/06/2020 23:30:44", "14,000000"], ["20/06/2020 23:30:44", "14,000000"], ["20/06/2020 23:30:44", "15,000000"], ["20/06/2020 23:30:44", "14,000000"], ["20/06/2020 23:30:44", "15,000000"], ["20/06/2020 23:30:44", "15,000000"], ["20/06/2020 23:30:44", "15,000000"], ["20/06/2020 23:30:44", "15,000000"], ["20/06/2020 23:30:44", "15,000000"], ["20/06/2020 23:30:44", "16,000000"], ["20/06/2020 23:30:44", "16,000000"], ["20/06/2020 23:30:44", "16,000000"], ["20/06/2020 23:30:44", "16,000000"], ["20/06/2020 23:30:44", "17,000000"], ["20/06/2020 23:30:44", "17,000000"], ["20/06/2020 23:30:44", "18,000000"], ["20/06/2020 23:30:44", "19,000000"], ["20/06/2020 23:30:44", "18,000000"], ["20/06/2020 23:30:44", "18,000000"], ["20/06/2020 23:30:44", "19,000000"], ["20/06/2020 23:30:44", "19,000000"], ["20/06/2020 23:30:44", "18,000000"], ["20/06/2020 23:30:44", "19,000000"], ["20/06/2020 23:30:44", "19,000000"], ["20/06/2020 23:30:44", "21,000000"], ["20/06/2020 23:30:44", "21,000000"], ["20/06/2020 23:30:44", "22,000000"], ["20/06/2020 23:30:44", "21,000000"], ["20/06/2020 23:30:44", "21,000000"], ["20/06/2020 23:30:44", "21,000000"], ["20/06/2020 23:30:44", "23,000000"], ["20/06/2020 23:30:44", "25,000000"], ["20/06/2020 23:30:44", "25,000000"], ["20/06/2020 23:30:44", "25,000000"], ["20/06/2020 23:30:44", "26,000000"], ["20/06/2020 23:30:44", "27,000000"], ["20/06/2020 23:30:44", "27,000000"], ["20/06/2020 23:30:44", "26,000000"], ["20/06/2020 23:30:44", "27,000000"], ["20/06/2020 23:30:44", "28,000000"], ["20/06/2020 23:30:44", "28,000000"], ["20/06/2020 23:30:44", "29,000000"], ["20/06/2020 23:30:44", "30,000000"], ["20/06/2020 23:30:44", "30,000000"], ["20/06/2020 23:30:44", "30,000000"], ["20/06/2020 23:30:44", "32,000000"], ["20/06/2020 23:30:44", "33,000000"], ["20/06/2020 23:30:44", "35,000000"], ["20/06/2020 23:30:44", "34,000000"], ["20/06/2020 23:30:44", "34,000000"], ["20/06/2020 23:30:44", "34,000000"], ["20/06/2020 23:30:44", "34,000000"], ["20/06/2020 23:30:44", "35,000000"], ["20/06/2020 23:30:44", "36,000000"], ["20/06/2020 23:30:44", "36,000000"], ["20/06/2020 23:30:44", "36,000000"], ["20/06/2020 23:30:44", "36,000000"], ["20/06/2020 23:30:44", "35,000000"], ["20/06/2020 23:30:44", "35,000000"], ["20/06/2020 23:30:44", "35,000000"], ["20/06/2020 23:30:44", "37,000000"], ["20/06/2020 23:30:44", "36,000000"], ["20/06/2020 23:30:44", "36,000000"], ["20/06/2020 23:30:44", "37,000000"], ["20/06/2020 23:30:44", "36,000000"], ["20/06/2020 23:30:44", "37,000000"], ["20/06/2020 23:30:44", "37,000000"], ["20/06/2020 23:30:44", "35,000000"], ["20/06/2020 23:30:44", "34,000000"], ["20/06/2020 23:30:44", "34,000000"], ["20/06/2020 23:30:44", "33,000000"], ["20/06/2020 23:30:44", "32,000000"], ["20/06/2020 23:30:44", "32,000000"], ["20/06/2020 23:30:44", "30,000000"], ["20/06/2020 23:30:44", "30,000000"], ["20/06/2020 23:30:44", "29,000000"], ["20/06/2020 23:30:44", "28,000000"], ["20/06/2020 23:30:44", "26,000000"], ["20/06/2020 23:30:44", "25,000000"], ["20/06/2020 23:30:44", "25,000000"], ["20/06/2020 23:30:44", "23,000000"], ["20/06/2020 23:30:44", "23,000000"], ["20/06/2020 23:30:44", "23,000000"], ["20/06/2020 23:30:44", "23,000000"], ["20/06/2020 23:30:44", "20,000000"], ["20/06/2020 23:30:44", "19,000000"], ["20/06/2020 23:30:44", "19,000000"], ["20/06/2020 23:30:44", "18,000000"], ["20/06/2020 23:30:44", "17,000000"], ["20/06/2020 23:30:44", "16,000000"], ["20/06/2020 23:30:44", "15,000000"], ["20/06/2020 23:30:44", "14,000000"], ["20/06/2020 23:30:44", "15,000000"], ["20/06/2020 23:30:44", "15,000000"], ["20/06/2020 23:30:44", "14,000000"], ["20/06/2020 23:30:44", "14,000000"], ["20/06/2020 23:30:44", "14,000000"], ["20/06/2020 23:30:44", "14,000000"], ["20/06/2020 23:30:44", "14,000000"], ["20/06/2020 23:30:44", "12,000000"], ["20/06/2020 23:30:44", "13,000000"], ["20/06/2020 23:30:44", "12,000000"], ["20/06/2020 23:30:44", "12,000000"], ["20/06/2020 23:30:44", "12,000000"], ["20/06/2020 23:30:44", "12,000000"], ["20/06/2020 23:30:44", "12,000000"], ["20/06/2020 23:30:44", "12,000000"], ["20/06/2020 23:30:44", "12,000000"], ["20/06/2020 23:30:44", "12,000000"], ["20/06/2020 23:30:44", "12,000000"], ["20/06/2020 23:30:44", "12,000000"], ["20/06/2020 23:30:44", "12,000000"], ["20/06/2020 23:30:44", "12,000000"], ["20/06/2020 23:30:44", "11,000000"], ["20/06/2020 23:30:44", "11,000000"], ["20/06/2020 23:30:44", "12,000000"], ["20/06/2020 23:30:44", "12,000000"], ["20/06/2020 23:30:44", "12,000000"], ["20/06/2020 23:30:44", "11,000000"], ["20/06/2020 23:30:44", "12,000000"], ["20/06/2020 23:30:44", "12,000000"], ["20/06/2020 23:30:44", "12,000000"], ["20/06/2020 23:30:44", "12,000000"], ["20/06/2020 23:30:44", "13,000000"], ["20/06/2020 23:30:44", "13,000000"], ["20/06/2020 23:30:44", "12,000000"], ["20/06/2020 23:30:44", "13,000000"], ["20/06/2020 23:30:44", "12,000000"], ["20/06/2020 23:30:44", "11,000000"], ["20/06/2020 23:30:44", "12,000000"], ["20/06/2020 23:30:44", "12,000000"], ["20/06/2020 23:30:44", "13,000000"], ["20/06/2020 23:30:44", "14,000000"], ["20/06/2020 23:30:44", "15,000000"], ["20/06/2020 23:30:44", "15,000000"], ["20/06/2020 23:30:44", "14,000000"], ["20/06/2020 23:30:44", "15,000000"], ["20/06/2020 23:30:44", "14,000000"], ["20/06/2020 23:30:44", "15,000000"], ["20/06/2020 23:30:44", "14,000000"], ["20/06/2020 23:30:44", "14,000000"], ["20/06/2020 23:30:44", "13,000000"], ["20/06/2020 23:30:44", "14,000000"], ["20/06/2020 23:30:44", "14,000000"], ["20/06/2020 23:30:44", "14,000000"], ["20/06/2020 23:30:44", "15,000000"], ["20/06/2020 23:30:44", "15,000000"], ["20/06/2020 23:30:44", "15,000000"], ["20/06/2020 23:30:44", "14,000000"], ["20/06/2020 23:30:44", "13,000000"], ["20/06/2020 23:30:44", "15,000000"], ["20/06/2020 23:30:44", "16,000000"], ["20/06/2020 23:30:44", "16,000000"], ["20/06/2020 23:30:44", "15,000000"], ["20/06/2020 23:30:44", "15,000000"], ["20/06/2020 23:30:44", "16,000000"], ["20/06/2020 23:30:44", "16,000000"], ["20/06/2020 23:30:44", "15,000000"], ["20/06/2020 23:30:44", "16,000000"], ["20/06/2020 23:30:44", "16,000000"], ["20/06/2020 23:30:44", "16,000000"], ["20/06/2020 23:30:44", "15,000000"], ["20/06/2020 23:30:44", "16,000000"], ["20/06/2020 23:30:44", "16,000000"], ["20/06/2020 23:30:44", "15,000000"], ["20/06/2020 23:30:44", "16,000000"], ["20/06/2020 23:30:44", "17,000000"], ["20/06/2020 23:30:44", "14,000000"], ["20/06/2020 23:30:44", "14,000000"], ["20/06/2020 23:30:44", "15,000000"], ["20/06/2020 23:30:44", "15,000000"], ["20/06/2020 23:30:44", "15,000000"], ["20/06/2020 23:30:44", "15,000000"], ["20/06/2020 23:30:44", "16,000000"], ["20/06/2020 23:30:44", "16,000000"], ["20/06/2020 23:30:44", "15,000000"], ["20/06/2020 23:30:44", "16,000000"], ["20/06/2020 23:30:44", "15,000000"], ["20/06/2020 23:30:44", "15,000000"], ["20/06/2020 23:30:44", "15,000000"], ["20/06/2020 23:30:44", "15,000000"], ["20/06/2020 23:30:44", "15,000000"], ["20/06/2020 23:30:44", "14,000000"], ["20/06/2020 23:30:44", "15,000000"], ["20/06/2020 23:30:44", "15,000000"], ["20/06/2020 23:30:44", "16,000000"], ["20/06/2020 23:30:44", "15,000000"], ["20/06/2020 23:30:44", "15,000000"], ["20/06/2020 23:30:44", "15,000000"], ["20/06/2020 23:30:44", "15,000000"], ["20/06/2020 23:30:44", "15,000000"], ["20/06/2020 23:30:44", "14,000000"], ["20/06/2020 23:30:44", "14,000000"], ["20/06/2020 23:30:44", "14,000000"], ["20/06/2020 23:30:44", "14,000000"], ["20/06/2020 23:30:44", "14,000000"], ["20/06/2020 23:30:44", "14,000000"], ["20/06/2020 23:30:44", "13,000000"], ["20/06/2020 23:30:44", "12,000000"], ["20/06/2020 23:30:44", "13,000000"], ["20/06/2020 23:30:44", "12,000000"], ["20/06/2020 23:30:44", "12,000000"], ["20/06/2020 23:30:44", "12,000000"], ["20/06/2020 23:30:44", "13,000000"], ["20/06/2020 23:30:44", "12,000000"], ["20/06/2020 23:30:44", "13,000000"], ["20/06/2020 23:30:44", "14,000000"], ["20/06/2020 23:30:44", "13,000000"], ["20/06/2020 23:30:44", "12,000000"], ["20/06/2020 23:30:44", "13,000000"], ["20/06/2020 23:30:44", "12,000000"], ["20/06/2020 23:30:44", "12,000000"], ["20/06/2020 23:30:44", "13,000000"], ["20/06/2020 23:30:44", "14,000000"], ["20/06/2020 23:30:44", "12,000000"], ["20/06/2020 23:30:44", "12,000000"], ["20/06/2020 23:30:44", "12,000000"], ["20/06/2020 23:30:44", "12,000000"], ["20/06/2020 23:30:44", "12,000000"], ["20/06/2020 23:30:44", "12,000000"], ["20/06/2020 23:30:44", "12,000000"], ["20/06/2020 23:30:44", "12,000000"], ["20/06/2020 23:30:44", "13,000000"], ["20/06/2020 23:30:44", "12,000000"], ["20/06/2020 23:30:44", "13,000000"], ["20/06/2020 23:30:44", "12,000000"], ["20/06/2020 23:30:44", "12,000000"], ["20/06/2020 23:30:44", "12,000000"], ["20/06/2020 23:30:44", "12,000000"], ["20/06/2020 23:30:44", "12,000000"], ["20/06/2020 23:30:44", "12,000000"], ["20/06/2020 23:30:44", "12,000000"], ["20/06/2020 23:30:44", "13,000000"], ["20/06/2020 23:30:44", "13,000000"], ["20/06/2020 23:30:44", "12,000000"], ["20/06/2020 23:30:44", "12,000000"], ["20/06/2020 23:30:44", "12,000000"], ["20/06/2020 23:30:44", "12,000000"], ["20/06/2020 23:30:44", "13,000000"], ["20/06/2020 23:30:44", "13,000000"], ["20/06/2020 23:30:44", "12,000000"], ["20/06/2020 23:30:44", "12,000000"], ["20/06/2020 23:30:44", "12,000000"], ["20/06/2020 23:30:44", "12,000000"], ["20/06/2020 23:30:44", "12,000000"], ["20/06/2020 23:30:44", "13,000000"], ["20/06/2020 23:30:44", "13,000000"], ["20/06/2020 23:30:44", "12,000000"], ["20/06/2020 23:30:44", "11,000000"], ["20/06/2020 23:30:44", "11,000000"], ["20/06/2020 23:30:44", "11,000000"], ["20/06/2020 23:30:45", "11,000000"], ["20/06/2020 23:30:45", "12,000000"], ["20/06/2020 23:30:45", "13,000000"], ["20/06/2020 23:30:45", "14,000000"], ["20/06/2020 23:30:45", "12,000000"], ["20/06/2020 23:30:45", "12,000000"], ["20/06/2020 23:30:45", "11,000000"], ["20/06/2020 23:30:45", "13,000000"], ["20/06/2020 23:30:45", "13,000000"], ["20/06/2020 23:30:45", "12,000000"], ["20/06/2020 23:30:45", "11,000000"], ["20/06/2020 23:30:45", "11,000000"], ["20/06/2020 23:30:45", "11,000000"], ["20/06/2020 23:30:45", "12,000000"], ["20/06/2020 23:30:45", "12,000000"], ["20/06/2020 23:30:45", "14,000000"], ["20/06/2020 23:30:45", "13,000000"], ["20/06/2020 23:30:45", "13,000000"], ["20/06/2020 23:30:45", "12,000000"], ["20/06/2020 23:30:45", "12,000000"], ["20/06/2020 23:30:45", "12,000000"], ["20/06/2020 23:30:45", "12,000000"], ["20/06/2020 23:30:45", "13,000000"], ["20/06/2020 23:30:45", "12,000000"], ["20/06/2020 23:30:45", "11,000000"], ["20/06/2020 23:30:45", "11,000000"], ["20/06/2020 23:30:45", "10,000000"], ["20/06/2020 23:30:45", "10,000000"], ["20/06/2020 23:30:45", "10,000000"], ["20/06/2020 23:30:45", "10,000000"], ["20/06/2020 23:30:45", "10,000000"], ["20/06/2020 23:30:45", "11,000000"], ["20/06/2020 23:30:45", "12,000000"], ["20/06/2020 23:30:45", "11,000000"], ["20/06/2020 23:30:45", "11,000000"], ["20/06/2020 23:30:45", "13,000000"], ["20/06/2020 23:30:45", "12,000000"], ["20/06/2020 23:30:45", "12,000000"], ["20/06/2020 23:30:45", "14,000000"], ["20/06/2020 23:30:45", "13,000000"], ["20/06/2020 23:30:45", "12,000000"], ["20/06/2020 23:30:45", "12,000000"], ["20/06/2020 23:30:45", "12,000000"], ["20/06/2020 23:30:45", "14,000000"], ["20/06/2020 23:30:45", "14,000000"], ["20/06/2020 23:30:45", "13,000000"], ["20/06/2020 23:30:45", "12,000000"], ["20/06/2020 23:30:45", "14,000000"], ["20/06/2020 23:30:45", "14,000000"], ["20/06/2020 23:30:45", "12,000000"], ["20/06/2020 23:30:45", "12,000000"], ["20/06/2020 23:30:45", "12,000000"], ["20/06/2020 23:30:45", "11,000000"], ["20/06/2020 23:30:45", "13,000000"], ["20/06/2020 23:30:45", "12,000000"], ["20/06/2020 23:30:45", "12,000000"], ["20/06/2020 23:30:45", "12,000000"], ["20/06/2020 23:30:45", "13,000000"], ["20/06/2020 23:30:45", "11,000000"], ["20/06/2020 23:30:45", "11,000000"], ["20/06/2020 23:30:45", "12,000000"], ["20/06/2020 23:30:45", "14,000000"], ["20/06/2020 23:30:45", "15,000000"], ["20/06/2020 23:30:45", "15,000000"], ["20/06/2020 23:30:45", "16,000000"], ["20/06/2020 23:30:45", "17,000000"], ["20/06/2020 23:30:45", "17,000000"], ["20/06/2020 23:30:45", "17,000000"], ["20/06/2020 23:30:45", "18,000000"], ["20/06/2020 23:30:45", "20,000000"], ["20/06/2020 23:30:45", "19,000000"], ["20/06/2020 23:30:45", "19,000000"], ["20/06/2020 23:30:45", "21,000000"], ["20/06/2020 23:30:45", "21,000000"], ["20/06/2020 23:30:45", "23,000000"], ["20/06/2020 23:30:45", "24,000000"], ["20/06/2020 23:30:45", "23,000000"], ["20/06/2020 23:30:45", "22,000000"], ["20/06/2020 23:30:45", "22,000000"], ["20/06/2020 23:30:45", "21,000000"], ["20/06/2020 23:30:45", "20,000000"], ["20/06/2020 23:30:45", "21,000000"], ["20/06/2020 23:30:45", "19,000000"], ["20/06/2020 23:30:45", "18,000000"], ["20/06/2020 23:30:45", "18,000000"], ["20/06/2020 23:30:45", "16,000000"], ["20/06/2020 23:30:45", "14,000000"], ["20/06/2020 23:30:45", "14,000000"], ["20/06/2020 23:30:45", "12,000000"], ["20/06/2020 23:30:45", "10,000000"], ["20/06/2020 23:30:45", "10,000000"], ["20/06/2020 23:30:45", "9,000000"], ["20/06/2020 23:30:45", "9,000000"], ["20/06/2020 23:30:45", "10,000000"], ["20/06/2020 23:30:45", "8,000000"], ["20/06/2020 23:30:45", "6,000000"], ["20/06/2020 23:30:45", "6,000000"], ["20/06/2020 23:30:45", "6,000000"], ["20/06/2020 23:30:45", "7,000000"], ["20/06/2020 23:30:45", "7,000000"], ["20/06/2020 23:30:45", "7,000000"], ["20/06/2020 23:30:45", "7,000000"], ["20/06/2020 23:30:45", "7,000000"], ["20/06/2020 23:30:45", "8,000000"], ["20/06/2020 23:30:45", "8,000000"], ["20/06/2020 23:30:45", "7,000000"], ["20/06/2020 23:30:45", "6,000000"], ["20/06/2020 23:30:45", "8,000000"], ["20/06/2020 23:30:45", "7,000000"], ["20/06/2020 23:30:45", "8,000000"], ["20/06/2020 23:30:45", "7,000000"], ["20/06/2020 23:30:45", "6,000000"], ["20/06/2020 23:30:45", "6,000000"], ["20/06/2020 23:30:45", "6,000000"], ["20/06/2020 23:30:45", "6,000000"], ["20/06/2020 23:30:45", "8,000000"], ["20/06/2020 23:30:45", "9,000000"], ["20/06/2020 23:30:45", "11,000000"], ["20/06/2020 23:30:45", "10,000000"], ["20/06/2020 23:30:45", "8,000000"], ["20/06/2020 23:30:45", "10,000000"], ["20/06/2020 23:30:45", "15,000000"], ["20/06/2020 23:30:45", "22,000000"], ["20/06/2020 23:30:45", "31,000000"], ["20/06/2020 23:30:45", "41,000000"], ["20/06/2020 23:30:45", "60,000000"], ["20/06/2020 23:30:45", "71,000000"], ["20/06/2020 23:30:45", "83,000000"], ["20/06/2020 23:30:45", "103,000000"], ["20/06/2020 23:30:45", "118,000000"], ["20/06/2020 23:30:45", "128,000000"], ["20/06/2020 23:30:45", "136,000000"], ["20/06/2020 23:30:45", "139,000000"], ["20/06/2020 23:30:45", "134,000000"], ["20/06/2020 23:30:45", "123,000000"], ["20/06/2020 23:30:45", "103,000000"], ["20/06/2020 23:30:45", "80,000000"], ["20/06/2020 23:30:45", "58,000000"], ["20/06/2020 23:30:45", "38,000000"], ["20/06/2020 23:30:45", "19,000000"], ["20/06/2020 23:30:45", "8,000000"], ["20/06/2020 23:30:45", "11,000000"], ["20/06/2020 23:30:45", "6,000000"], ["20/06/2020 23:30:45", "5,000000"], ["20/06/2020 23:30:45", "3,000000"], ["20/06/2020 23:30:45", "0,000000"], ["20/06/2020 23:30:45", "1,000000"], ["20/06/2020 23:30:45", "0,000000"], ["20/06/2020 23:30:45", "3,000000"], ["20/06/2020 23:30:45", "4,000000"], ["20/06/2020 23:30:45", "3,000000"], ["20/06/2020 23:30:45", "5,000000"], ["20/06/2020 23:30:45", "6,000000"], ["20/06/2020 23:30:45", "7,000000"], ["20/06/2020 23:30:45", "9,000000"], ["20/06/2020 23:30:45", "11,000000"], ["20/06/2020 23:30:45", "11,000000"], ["20/06/2020 23:30:45", "10,000000"], ["20/06/2020 23:30:45", "10,000000"], ["20/06/2020 23:30:45", "10,000000"], ["20/06/2020 23:30:45", "10,000000"], ["20/06/2020 23:30:45", "10,000000"], ["20/06/2020 23:30:45", "12,000000"], ["20/06/2020 23:30:45", "10,000000"], ["20/06/2020 23:30:45", "11,000000"], ["20/06/2020 23:30:45", "10,000000"], ["20/06/2020 23:30:45", "11,000000"], ["20/06/2020 23:30:45", "11,000000"], ["20/06/2020 23:30:45", "12,000000"], ["20/06/2020 23:30:45", "10,000000"], ["20/06/2020 23:30:45", "9,000000"], ["20/06/2020 23:30:45", "12,000000"], ["20/06/2020 23:30:45", "10,000000"], ["20/06/2020 23:30:45", "12,000000"], ["20/06/2020 23:30:45", "11,000000"], ["20/06/2020 23:30:45", "12,000000"], ["20/06/2020 23:30:45", "11,000000"], ["20/06/2020 23:30:45", "10,000000"], ["20/06/2020 23:30:45", "10,000000"], ["20/06/2020 23:30:45", "11,000000"], ["20/06/2020 23:30:45", "11,000000"], ["20/06/2020 23:30:45", "11,000000"], ["20/06/2020 23:30:45", "12,000000"], ["20/06/2020 23:30:46", "11,000000"], ["20/06/2020 23:30:46", "12,000000"], ["20/06/2020 23:30:46", "12,000000"], ["20/06/2020 23:30:46", "11,000000"], ["20/06/2020 23:30:46", "10,000000"], ["20/06/2020 23:30:46", "11,000000"], ["20/06/2020 23:30:46", "11,000000"], ["20/06/2020 23:30:46", "10,000000"], ["20/06/2020 23:30:46", "11,000000"], ["20/06/2020 23:30:46", "11,000000"], ["20/06/2020 23:30:46", "12,000000"], ["20/06/2020 23:30:46", "11,000000"], ["20/06/2020 23:30:46", "12,000000"], ["20/06/2020 23:30:46", "12,000000"], ["20/06/2020 23:30:46", "13,000000"], ["20/06/2020 23:30:46", "13,000000"], ["20/06/2020 23:30:46", "12,000000"], ["20/06/2020 23:30:46", "12,000000"], ["20/06/2020 23:30:46", "12,000000"], ["20/06/2020 23:30:46", "13,000000"], ["20/06/2020 23:30:46", "13,000000"], ["20/06/2020 23:30:46", "13,000000"], ["20/06/2020 23:30:46", "14,000000"], ["20/06/2020 23:30:46", "14,000000"], ["20/06/2020 23:30:46", "15,000000"], ["20/06/2020 23:30:46", "16,000000"], ["20/06/2020 23:30:46", "15,000000"], ["20/06/2020 23:30:46", "15,000000"], ["20/06/2020 23:30:46", "16,000000"], ["20/06/2020 23:30:46", "14,000000"], ["20/06/2020 23:30:46", "15,000000"], ["20/06/2020 23:30:46", "16,000000"], ["20/06/2020 23:30:46", "17,000000"], ["20/06/2020 23:30:46", "18,000000"], ["20/06/2020 23:30:46", "17,000000"], ["20/06/2020 23:30:46", "16,000000"], ["20/06/2020 23:30:46", "17,000000"], ["20/06/2020 23:30:46", "17,000000"], ["20/06/2020 23:30:46", "18,000000"], ["20/06/2020 23:30:46", "18,000000"], ["20/06/2020 23:30:46", "19,000000"], ["20/06/2020 23:30:46", "19,000000"], ["20/06/2020 23:30:46", "20,000000"], ["20/06/2020 23:30:46", "19,000000"], ["20/06/2020 23:30:46", "20,000000"], ["20/06/2020 23:30:46", "21,000000"], ["20/06/2020 23:30:46", "20,000000"], ["20/06/2020 23:30:46", "20,000000"], ["20/06/2020 23:30:46", "21,000000"], ["20/06/2020 23:30:46", "22,000000"], ["20/06/2020 23:30:46", "23,000000"], ["20/06/2020 23:30:46", "23,000000"], ["20/06/2020 23:30:46", "25,000000"], ["20/06/2020 23:30:46", "25,000000"], ["20/06/2020 23:30:46", "26,000000"], ["20/06/2020 23:30:46", "25,000000"], ["20/06/2020 23:30:46", "25,000000"], ["20/06/2020 23:30:46", "26,000000"], ["20/06/2020 23:30:46", "27,000000"], ["20/06/2020 23:30:46", "27,000000"], ["20/06/2020 23:30:46", "28,000000"], ["20/06/2020 23:30:46", "29,000000"], ["20/06/2020 23:30:46", "30,000000"], ["20/06/2020 23:30:46", "30,000000"], ["20/06/2020 23:30:46", "31,000000"], ["20/06/2020 23:30:46", "31,000000"], ["20/06/2020 23:30:46", "30,000000"], ["20/06/2020 23:30:46", "31,000000"], ["20/06/2020 23:30:46", "32,000000"], ["20/06/2020 23:30:46", "33,000000"], ["20/06/2020 23:30:46", "33,000000"], ["20/06/2020 23:30:46", "35,000000"], ["20/06/2020 23:30:46", "35,000000"], ["20/06/2020 23:30:46", "34,000000"], ["20/06/2020 23:30:46", "36,000000"], ["20/06/2020 23:30:46", "36,000000"], ["20/06/2020 23:30:46", "37,000000"], ["20/06/2020 23:30:46", "37,000000"], ["20/06/2020 23:30:46", "37,000000"], ["20/06/2020 23:30:46", "38,000000"], ["20/06/2020 23:30:46", "37,000000"], ["20/06/2020 23:30:46", "36,000000"], ["20/06/2020 23:30:46", "37,000000"], ["20/06/2020 23:30:46", "38,000000"], ["20/06/2020 23:30:46", "38,000000"], ["20/06/2020 23:30:46", "38,000000"], ["20/06/2020 23:30:46", "36,000000"], ["20/06/2020 23:30:46", "36,000000"], ["20/06/2020 23:30:46", "36,000000"], ["20/06/2020 23:30:46", "37,000000"], ["20/06/2020 23:30:46", "35,000000"], ["20/06/2020 23:30:46", "35,000000"], ["20/06/2020 23:30:46", "35,000000"], ["20/06/2020 23:30:46", "35,000000"], ["20/06/2020 23:30:46", "32,000000"], ["20/06/2020 23:30:46", "33,000000"], ["20/06/2020 23:30:46", "32,000000"], ["20/06/2020 23:30:46", "31,000000"], ["20/06/2020 23:30:46", "30,000000"], ["20/06/2020 23:30:46", "29,000000"], ["20/06/2020 23:30:46", "28,000000"], ["20/06/2020 23:30:46", "27,000000"], ["20/06/2020 23:30:46", "27,000000"], ["20/06/2020 23:30:46", "26,000000"], ["20/06/2020 23:30:46", "24,000000"], ["20/06/2020 23:30:46", "23,000000"], ["20/06/2020 23:30:47", "22,000000"], ["20/06/2020 23:30:47", "20,000000"], ["20/06/2020 23:30:47", "21,000000"], ["20/06/2020 23:30:47", "20,000000"], ["20/06/2020 23:30:47", "18,000000"], ["20/06/2020 23:30:47", "19,000000"], ["20/06/2020 23:30:47", "19,000000"], ["20/06/2020 23:30:47", "16,000000"], ["20/06/2020 23:30:47", "17,000000"], ["20/06/2020 23:30:47", "16,000000"], ["20/06/2020 23:30:47", "16,000000"], ["20/06/2020 23:30:47", "17,000000"], ["20/06/2020 23:30:47", "16,000000"], ["20/06/2020 23:30:47", "16,000000"], ["20/06/2020 23:30:47", "14,000000"], ["20/06/2020 23:30:47", "14,000000"], ["20/06/2020 23:30:47", "14,000000"], ["20/06/2020 23:30:47", "13,000000"], ["20/06/2020 23:30:47", "13,000000"], ["20/06/2020 23:30:47", "13,000000"], ["20/06/2020 23:30:47", "13,000000"], ["20/06/2020 23:30:47", "12,000000"], ["20/06/2020 23:30:47", "15,000000"], ["20/06/2020 23:30:47", "14,000000"], ["20/06/2020 23:30:47", "14,000000"], ["20/06/2020 23:30:47", "14,000000"], ["20/06/2020 23:30:47", "14,000000"], ["20/06/2020 23:30:47", "15,000000"], ["20/06/2020 23:30:47", "11,000000"], ["20/06/2020 23:30:47", "12,000000"], ["20/06/2020 23:30:47", "13,000000"], ["20/06/2020 23:30:47", "12,000000"], ["20/06/2020 23:30:47", "13,000000"], ["20/06/2020 23:30:47", "13,000000"], ["20/06/2020 23:30:47", "13,000000"], ["20/06/2020 23:30:47", "14,000000"], ["20/06/2020 23:30:47", "13,000000"], ["20/06/2020 23:30:47", "12,000000"], ["20/06/2020 23:30:47", "12,000000"], ["20/06/2020 23:30:47", "13,000000"], ["20/06/2020 23:30:47", "12,000000"], ["20/06/2020 23:30:47", "13,000000"], ["20/06/2020 23:30:47", "12,000000"], ["20/06/2020 23:30:47", "13,000000"], ["20/06/2020 23:30:47", "12,000000"], ["20/06/2020 23:30:47", "14,000000"], ["20/06/2020 23:30:47", "14,000000"], ["20/06/2020 23:30:47", "14,000000"], ["20/06/2020 23:30:47", "12,000000"], ["20/06/2020 23:30:47", "12,000000"], ["20/06/2020 23:30:47", "14,000000"], ["20/06/2020 23:30:47", "14,000000"], ["20/06/2020 23:30:47", "14,000000"], ["20/06/2020 23:30:47", "15,000000"], ["20/06/2020 23:30:47", "15,000000"], ["20/06/2020 23:30:47", "15,000000"], ["20/06/2020 23:30:47", "14,000000"], ["20/06/2020 23:30:47", "14,000000"], ["20/06/2020 23:30:47", "14,000000"], ["20/06/2020 23:30:47", "14,000000"], ["20/06/2020 23:30:47", "13,000000"], ["20/06/2020 23:30:47", "14,000000"], ["20/06/2020 23:30:47", "14,000000"], ["20/06/2020 23:30:47", "13,000000"], ["20/06/2020 23:30:47", "12,000000"], ["20/06/2020 23:30:47", "16,000000"], ["20/06/2020 23:30:47", "14,000000"], ["20/06/2020 23:30:47", "14,000000"], ["20/06/2020 23:30:47", "14,000000"], ["20/06/2020 23:30:47", "14,000000"], ["20/06/2020 23:30:47", "12,000000"], ["20/06/2020 23:30:47", "14,000000"], ["20/06/2020 23:30:47", "13,000000"], ["20/06/2020 23:30:47", "12,000000"], ["20/06/2020 23:30:47", "12,000000"], ["20/06/2020 23:30:47", "14,000000"], ["20/06/2020 23:30:47", "14,000000"], ["20/06/2020 23:30:47", "13,000000"], ["20/06/2020 23:30:47", "15,000000"], ["20/06/2020 23:30:47", "13,000000"], ["20/06/2020 23:30:47", "12,000000"], ["20/06/2020 23:30:47", "11,000000"], ["20/06/2020 23:30:47", "12,000000"], ["20/06/2020 23:30:47", "12,000000"], ["20/06/2020 23:30:47", "13,000000"], ["20/06/2020 23:30:47", "14,000000"], ["20/06/2020 23:30:47", "14,000000"], ["20/06/2020 23:30:47", "14,000000"], ["20/06/2020 23:30:47", "14,000000"], ["20/06/2020 23:30:47", "13,000000"], ["20/06/2020 23:30:47", "14,000000"], ["20/06/2020 23:30:47", "12,000000"], ["20/06/2020 23:30:47", "13,000000"], ["20/06/2020 23:30:47", "13,000000"], ["20/06/2020 23:30:47", "13,000000"], ["20/06/2020 23:30:47", "13,000000"], ["20/06/2020 23:30:47", "14,000000"], ["20/06/2020 23:30:47", "14,000000"]]
  in  "Reset":bool
  in  "ON/OFF":bool=TRUE caption="Enable"
  out "Amplitude ECG\n    Amplifiée":i32
  out "FFT Signal filtré":dynamicdata(graph)=[{"t0"=timestamp(0 s since 1904-01-01), "dt"=1.0, "Y"=array[500 elements], "attributes"=variant("NI_ChannelName"=variant(string "Filtered (FFT - (Peak))"), "NI_OriginalChannelName"=variant(string "Filtered"))}]
  out "FFT Signal bruité":cluster{"f0":dbl, "df":dbl, "magnitude":dbl[]}(graph)={"f0"=0.0, "df"=1.0, "magnitude"=[18.30335548669678, 12.942426783111301, 2.298414330584108e-15, 2.064487798912609e-15, 3.9009779793918365e-15, 1.7996397492373118e-15, 3.811209746290715e-15, 1.3270039887675485e-16, 2.2396703603609874e-15, 3.1011395139172054e-15, 3.0014745525010715e-15, 1.4814403090970613e-15, 7.149350691879732e-16, 2.4472821380876606e-15, 9.379270066490015e-16, 1.2213848980311172e-15, 1.1489345785156068e-15, 2.313842202999342e-16, 1.434049379395675e-15, 2.3247785314131202e-15, 6.099461933567887e-15, 5.587331311413288e-15, 2.3193628632818355e-15, 2.143665310808698e-15, 1.1900649248884933e-15, 2.9728504265311373e-15, 6.714376355298734e-16, 1.783813554981419e-15, 1.0220327998750545e-15, 9.095982761708397e-16, 3.906295794904873e-15, 7.081241054738808e-16, 1.4836796675447045e-15, 3.316336446284211e-16, 1.475847067584821e-15, 3.4577982007013015e-15, 1.5894999279273397e-15, 2.4646828831138986e-15, 6.379989319460043e-16, 6.5869726717355785e-15, 2.3234225694711845e-15, 1.028408258340696e-14, 5.629872383842067e-15, 4.972567949232478e-15, 6.018726269435896e-15, 6.7201335727914056e-15, 8.189196647759912e-15, 5.636004458635832e-15, 3.708827480563746e-14, 110.00000000000006, 220.00000000000003, 110.00000000000007, 3.8463296068500826e-14, 3.276738469371446e-15, 1.0039700221049546e-14, 4.754515205992131e-15, 5.446547934417983e-15, 5.351640329917916e-15, 5.505606109229405e-15, 7.229939797366805e-15, 2.1727138245347916e-15, 4.787090999608993e-15, 1.708285034408051e-15, 3.0083337929439968e-15, 3.7013960228806144e-15, 3.918396874832064e-15, 2.94460294202862e-15, 1.1441865074316665e-15, 2.6203402282709584e-15, 2.740185132171002e-15, 5.193416091696026e-15, 2.8464646776479923e-15, 1.4545144398398281e-15, 1.3269927938616203e-15, 1.8813471025583246e-15, 1.9779719729217922e-15, 2.014398898003429e-15, 3.9609768952506377e-16, 9.596752167080804e-16, 5.8788996449906664e-15, 5.656250896240177e-15, 2.2671652541380375e-15, 1.880944406697374e-15, 3.2472273139550577e-15, 7.968565615800995e-16, 1.7842366940026216e-15, 1.3359842157516307e-15, 8.847072696031935e-16, 1.445138184543323e-15, 4.710213164040685e-15, 3.968920089877797e-15, 3.886912166993248e-15, 1.679140131659646e-15, 1.7586116546054594e-16, 3.6553320720970256e-15, 1.0294147007608229e-16, 3.403234182921681e-15, 4.397030778853802e-16, 1.6676474044114098e-15, 1.814183900203789e-15, 3.4700865309060302e-15, 3.3799772727887265e-15, 2.0197303479299573e-15, 2.190311067802262e-15, 1.3448765375118144e-16, 1.1827856603830658e-15, 2.3215832908161215e-15, 1.8946741115018962e-15, 1.8897155687041945e-15, 4.8174648083072535e-15, 1.909261685897886e-15, 4.4228781869126076e-15, 7.286429862260532e-16, 1.7811174182214284e-15, 1.497809551924363e-15, 3.3472269772784298e-15, 1.7260783254600674e-15, 1.0066842851233621e-15, 2.160245449682692e-15, 6.6321243415847066e-15, 6.527019122084488e-15, 6.037089773495911e-15, 1.7603050259108023e-15, 7.156561516981031e-16, 1.6849736328791088e-15, 1.0712864163587488e-15, 1.8341810137303445e-15, 1.5561775574608696e-15, 1.6801952258718621e-15, 4.5202812787639945e-15, 3.6588162633371645e-15, 5.6966104887261884e-15, 2.922851962453663e-15, 1.9286875071733097e-15, 1.78840465601051e-15, 9.46007947058019e-16, 1.0979816925491725e-15, 3.0374329705996585e-15, 7.191456059178644e-16, 3.280234673954272e-15, 3.2650911072658375e-15, 4.418966391878891e-15, 6.008813876641293e-16, 3.704172604186971e-15, 1.9515567694318248e-15, 3.1412315800865732e-15, 4.424752822765374e-16, 2.001325689609228e-15, 8.949605470403224e-16, 7.702786210914862e-15, 7.347004936101772e-15, 8.191773960843652e-15, 1.13355824185465e-15, 2.437623344514476e-15, 5.488140128417641e-16, 9.731515269237607e-16, 1.6065975896306107e-15, 1.823454696433862e-15, 1.983585006162922e-15, 1.928797285036307e-15, 2.319568640034727e-15, 3.235689510062392e-15, 1.2511407166222289e-15, 1.6202356266921781e-15, 2.7195425352933596e-15, 3.100525549832563e-15, 1.877144700553242e-15, 1.6150063034038907e-15, 6.339114453731536e-16, 4.521528050085867e-15, 7.001657527523632e-15, 6.434326247960783e-15, 1.1237660100317113e-15, 2.3530015130234766e-15, 3.0603481398784307e-15, 1.7452701833010638e-15, 2.1392803597630383e-15, 9.625455727195246e-16, 2.192058582935939e-15, 4.9351575972455146e-15, 4.1326546117209306e-15, 3.449265227217328e-15, 5.045928610169757e-16, 6.088683608832926e-16, 2.44075382720278e-15, 2.0440157794339363e-15, 5.213362606336637e-16, 1.6591059993461108e-15, 1.633408853852595e-15, 2.637739301704842e-15, 3.186101852877381e-15, 1.9937365978854553e-15, 2.0573733647317068e-15, 1.5243135209608433e-15, 1.1790701458355936e-15, 2.240052690941721e-15, 1.3650162500941483e-15, 1.831690507864838e-15, 7.925340236299343e-16, 9.877791665834495e-16, 7.395006073002675e-15, 1.6189133488885992e-15, 9.95304231098068e-16, 4.0952376703839573e-16, 1.0240891799414464e-15, 7.233486415905968e-16, 3.482341134613188e-15, 6.239585690744641e-16, 1.52392185985271e-15, 3.609633110387839e-15, 2.8494415438303785e-15, 6.410743812208006e-15, 1.0500317355834158e-15, 2.3816402448569962e-15, 3.641460188069512e-15, 3.6525332773374876e-15, 2.885521341786495e-15, 1.1262216832218565e-15, 2.0368028676060803e-15, 4.286460167525576e-15, 6.7473218020094266e-15, 1.8021632066080155e-15, 2.9081342085771644e-16, 4.876004553454327e-16, 1.7665393648272651e-15, 2.736207009042221e-15, 1.4894205449628245e-15, 3.1414088558691375e-16, 2.876297139547007e-15, 7.008934335674629e-15, 5.26614839117052e-15, 6.578491689575094e-15, 3.662405979875157e-15, 2.594480921773983e-15, 1.4591378230863081e-15, 8.9083947888996e-16, 1.4831486245602517e-16, 1.5394434588935104e-15, 1.944250566924831e-16, 9.02240516161726e-16, 3.1367196209087815e-15, 1.2917762458954774e-15, 1.2437388682167813e-15, 2.0017990088804057e-15, 2.108356533647104e-15, 1.063541418587842e-15, 1.0952836434503114e-15, 6.338733563621039e-16, 2.2951185530061986e-15, 1.366046466748754e-14, 2.404975948528397e-14, 2.5850419188932305e-14, 8.538253541282803e-16, 1.2665283699713174e-15, 2.1436247507280143e-15, 2.9846461438229426e-15, 2.42072287843976e-15, 1.1115265282206234e-15, 2.0063831827547136e-15, 1.902921674383389e-15, 1.7498445934770145e-15, 2.872500023982007e-15, 4.903696387302726e-16, 2.542320395621183e-15, 1.4686836712351714e-15, 2.5186795004380945e-15, 9.028745332263703e-16, 9.234067099469372e-16, 2.4449352271393063e-15, 4.1272385992216616e-15, 6.48124553159418e-15, 6.937183714012712e-15, 2.3746667940006728e-15, 2.25044688384175e-15, 2.188521635104934e-15, 8.494259028477513e-16, 1.7438764335463182e-15, 1.075563499376501e-15, 1.3375270650194886e-15, 4.119939553716745e-15, 4.04487341517876e-15, 1.9458605353939654e-15, 1.6988739932859329e-15, 1.319469219777166e-15, 1.6130210841851362e-15, 3.532768959418546e-16, 1.5260500582231802e-15, 3.089548405340069e-15, 1.013935058290211e-15, 3.044837399145386e-15, 6.386166122684988e-16, 2.963941203512415e-15, 1.1474769009676996e-15, 6.993456471169242e-16, 2.656510258587479e-15, 2.3509028771127366e-15, 2.8258799923926657e-15, 3.6912204832772e-15, 2.8943653633294898e-15, 4.2864806957015104e-15, 1.2649587616956307e-14, 3.943815516254455e-15, 1.5568103297991719e-15, 4.80004355829865e-15, 2.881315275752287e-15, 2.8067087625840946e-15, 3.696633914224078e-15, 2.0453291812595077e-15, 2.2864886322449846e-15, 3.84885529318777e-15, 3.1802262057479564e-15, 3.6890202042358085e-15, 2.816888806893341e-16, 1.9566979295809713e-15, 1.847709400883879e-15, 2.050578420889432e-15, 1.6922117428269866e-15, 7.770560272543428e-16, 1.8495081556718317e-15, 1.4007036790827332e-15, 7.607329905961026e-15, 1.923385227410138e-15, 3.2259794090576557e-15, 2.447451112740395e-15, 4.4267487193329714e-15, 2.6148994396387944e-15, 2.335946052620763e-15, 1.2796221373344984e-15, 2.437743483801776e-15, 2.2282629638720416e-15, 7.353322390671361e-15, 4.276750637360401e-15, 2.3055266831263375e-16, 5.188951099747345e-16, 1.6879187299936125e-15, 5.86878266596437e-16, 6.925882392021458e-16, 1.6929281091894908e-15, 4.695241995653485e-16, 1.163676530692102e-15, 1.7102228787186494e-15, 1.0260540714028103e-15, 2.7897423075480916e-15, 1.0358095616068344e-15, 2.0508616641488365e-15, 3.6021178275099154e-16, 2.2403016295641585e-15, 4.503233437508441e-16, 2.5060123534624054e-15, 1.9176618638794936e-14, 1.5361494286816654e-14, 2.4095894994300152e-14, 1.6077434121896788e-15, 1.6200954425487312e-15, 2.1331805455212552e-15, 2.169839242420686e-15, 1.3746550959642541e-15, 1.3766129453777287e-15, 9.434548555506966e-16, 2.8734622711149815e-15, 7.999119057179207e-16, 8.846269164962903e-16, 1.4343955109144762e-15, 2.8657953823010506e-15, 1.4698008781345163e-15, 1.3719194906523912e-15, 1.542406984516754e-15, 2.838332052000218e-16, 2.0043628414878386e-15, 2.822533591377534e-15, 5.660674715307447e-15, 3.7686840708062336e-15, 1.2686524908167753e-15, 1.8792926466604415e-15, 9.640772031147875e-16, 1.8378261550425524e-15, 4.514185014002635e-16, 1.6800726790117614e-15, 2.9253931621756167e-15, 1.6966166523591587e-15, 5.236109158564861e-15, 1.314254042181566e-15, 2.955338282460582e-15, 5.861721620807671e-16, 2.1204577166979586e-15, 1.8547877938866853e-15, 1.4511546593944839e-15, 7.58572283502388e-16, 1.8062026620495044e-15, 3.1947102729366733e-15, 1.0104233014847042e-15, 2.246460221821866e-15, 6.549735185689737e-16, 1.2177862984662904e-15, 1.4941968188098884e-15, 6.289488823369237e-16, 3.3170813810084017e-15, 4.467765460000119e-15, 3.293728651695929e-15, 4.088033244584985e-15, 9.180426356611234e-15, 4.693021312818411e-15, 2.2389008798556412e-15, 4.193058978707965e-15, 1.6414911587044795e-15, 2.599633045065466e-15, 1.3137656346147068e-15, 2.467619493628327e-15, 8.399794637816032e-16, 2.204499199879853e-15, 1.9813383761494254e-15, 1.6159120473375164e-15, 1.2542925021469852e-15, 2.4323315603706147e-15, 1.330352651557897e-15, 2.341646675684958e-15, 6.446643292614642e-16, 7.145389539414783e-16, 1.2990555809041216e-15, 1.5723145202086236e-15, 8.592565216685965e-15, 2.280411761212714e-15, 3.2174057149596962e-15, 3.3533840579346006e-15, 4.918435798203131e-15, 2.9143575874673786e-15, 4.135126423319217e-15, 2.311422916425273e-15, 2.985643183657603e-15, 2.5840352968386984e-15, 7.37151415199944e-15, 3.5153887270673216e-15, 9.174797672096644e-16, 3.395513847690804e-16, 3.328662656905155e-15, 1.884293384152324e-15, 3.3357901095393235e-15, 1.895838423088303e-15, 2.6871422012169277e-15, 3.02309230423357e-15, 6.358006542620843e-16, 4.548669356666733e-15, 3.9279627385310325e-15, 4.407350134147068e-16, 1.4726232124235951e-15, 4.855808255492631e-16, 2.0216060903791578e-15, 1.2911137017483849e-15, 2.909239593324731e-16, 1.423529538790937e-13, 2.6939669292584897e-13, 1.475092743294719e-13, 2.430177199341669e-15, 2.0867411670926893e-15, 2.567982521157395e-15, 1.393243359918336e-15, 2.251020112196401e-15, 2.5892256963984718e-15, 2.8323074631501734e-15, 1.08598113565163e-15, 2.696270374179431e-16, 2.35675897574896e-15, 2.7560824281128743e-15, 9.154044970654436e-16, 3.03854696901392e-15, 2.153791383096155e-15, 2.288566037330859e-15, 7.376867995407741e-16, 1.1841595490625133e-15, 1.9359149191259802e-15, 6.562025022987788e-15, 2.5312275643111816e-15, 2.8960470381164853e-15, 7.728912866261049e-16, 2.3608065429024433e-15, 1.8578203544179932e-15, 2.137253140190377e-15, 4.0972965676816187e-16, 2.0873456706275636e-15, 5.041815543949071e-15, 7.121570450899988e-15, 3.079618547444899e-15, 8.760001209995964e-16, 6.554241264841169e-16, 3.3128914199427755e-15, 1.3660512722945246e-15, 2.9998787363005192e-15, 1.4736435601530969e-16, 1.4138665741388533e-15, 2.8279341536913612e-15, 1.7280866301054357e-15, 2.489330421864404e-15, 7.626723280940632e-16, 3.1793460481439186e-16, 9.469913262754883e-16, 1.7563378627958704e-15, 2.7567771753918244e-15, 2.3681082234407214e-15, 2.929005119442018e-15, 1.8459629853848063e-15]}
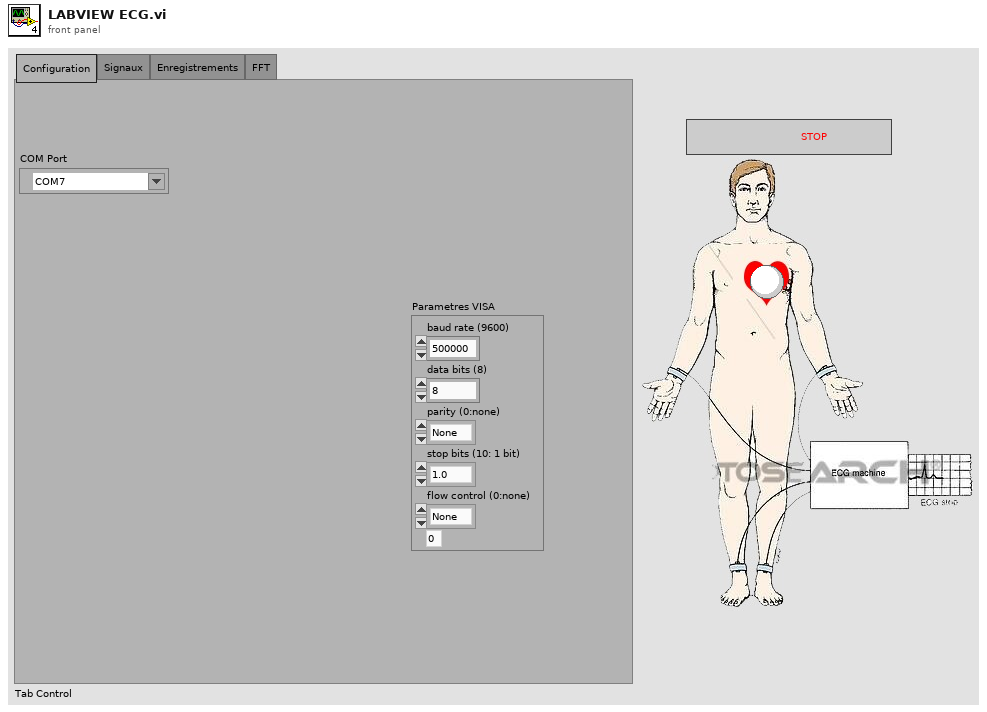
[diagram p1: front panel]
types:
  T1 = enum32{"Configuration", "Signaux", "Enregistrements", "FFT"}
  T2 = cluster{"baud rate (9600)":u32, "data bits (8)":u16, "parity (0:none)":enum16{"None", "Odd", "Even", "Mark", "Space"}, "stop bits (10: 1 bit)":u16, "flow control (0:none)":u16}
  T3 = typedef "Select Event Type.ctl" = u32
  T4 = cluster{"averaging mode":u16, "weighting mode":u16, "number of averages":u32}
  T5 = cluster{"dB On (F)":bool, "unwrap phase (F)":bool, "convert to degree (F)":bool}
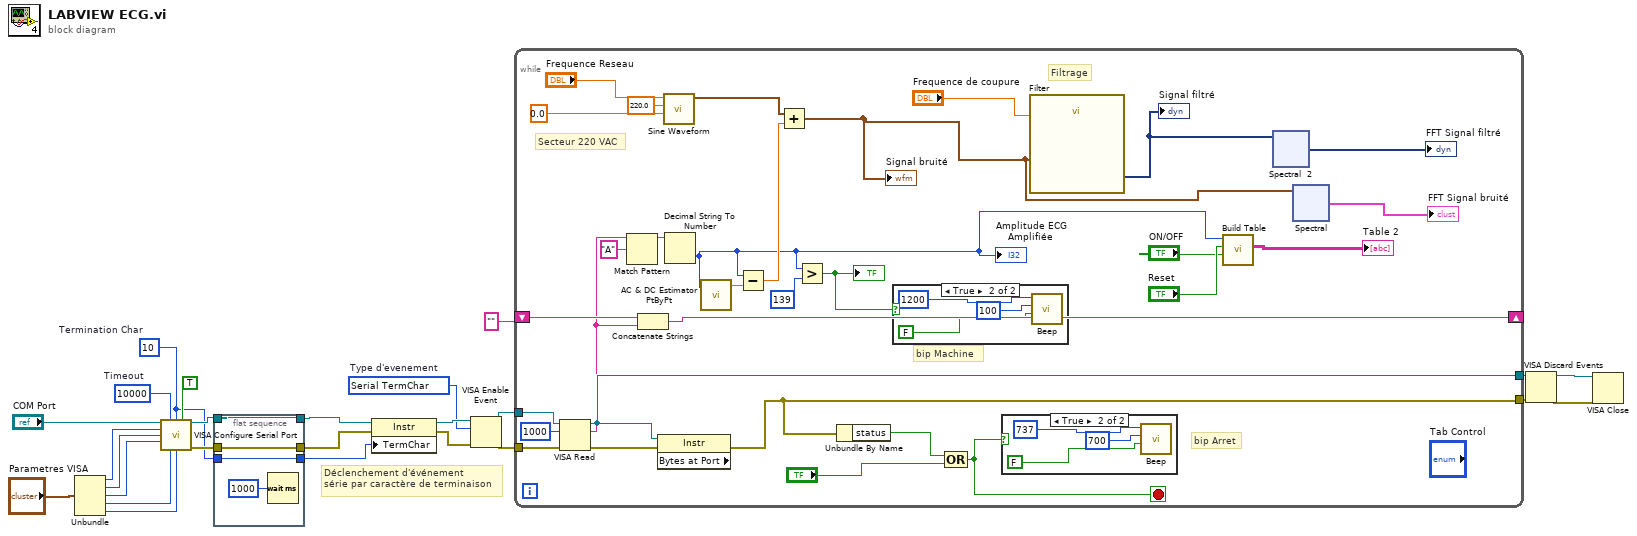
[diagram p0: block diagram]
diagram:
  w10 = T3 1073684516 items=["Service Request"=1073684491, "Trigger"=3221168138, "Clear"=1073684493, "VXI Signal"=1073684512, "VXI/VME Interrupt"=3221168161, "VXI/VME Sysfail"=1073684509, "VXI/VME Sysreset"=1073684510, "GPIB CIC"=1073684498, "GPIB Talk"=1073684499, "GPIB Listen"=1073684500, "PXI Interrupt"=1073684514, "Serial Break"=1073684515, "Serial TermChar"=1073684516, "Serial CTS"=1073684521, "Serial DSR"=1073684522, "Serial DCD"=1073684524, "Serial RI"=1073684526, "Serial Character"=1073684533, "USB Interrupt"=1073684535, "All Enabled"=1073709055]  # Type d'evenement
  w2 = u8 10  # Termination Char
  w18 = u32 10000  # Timeout
  # "Déclenchement d'événement\nsérie par caractère de terminaison"
  n1 = Unbundle("Parametres VISA") -> ("baud rate (9600)"=w23:u32, "data bits (8)"=w22:u16, "parity (0:none)"=w21:enum16{"None", "Odd", "Even", "Mark", "Space"}, "stop bits (10: 1 bit)"=w20:u16, "flow control (0:none)"=w19:u16)
  n2 = call-poly "VISA Configure Serial Port"("VISA resource name"="COM Port", "timeout (10sec)"=w18, "termination char\n(0xA = '\\n' = LF)"=w2, "Enable Termination\nChar (T)"=TRUE ("Enable Termination\nChar (T)"), "baud rate (9600)"=w23, "data bits (8)"=w22, "parity (0:none)"=w21, "stop bits (10: 1 bit)"=w20, "flow control (0:none)"=w19) -> ("VISA resource name out"=w3:refnum<visa-resource-name>, "error out"=w5:errorcluster)  [unwired: 5 in]
  n3 = flat-sequence {
    tunnel: [w28] -> w6
    tunnel: w5 -> [w28]
    tunnel: [w27] -> w4
    tunnel: w3 -> [w27]
    tunnel: w2 -> [w26]
    tunnel: [w26] -> w1
    frame #0 {
      n4 = Wait (ms)(milliseconds to wait=u32 1000) -> ()  [unwired: 1 out]
    }
  }
  n5 = property class="Instr"(reference=w4, error in=w6, "TermChar"=w1) -> (reference out=w12:refnum<visa-resource-name>, error out=w11:errorcluster)
  n6 = VISA Enable Event(8:w11, 10:w10, 11:w12) -> (0:w8:errorcluster, 3:w9:refnum<visa-resource-name>)  [unwired: 1 in]
  n7 = while {
    tunnel: w9 -> [w58]
    tunnel: w8 -> [w57]
    tunnel: [w54] -> w14
    tunnel: [w44] -> w15
    shift-right: [w52] -> _
    shift-left: "" -> [w53]
    stop <- w49 stop-if-true
    # "Filtrage"
    # "bip Arret"
    # "bip Machine"
    # "Secteur 220 VAC"
    n8 = VISA Read(VISA resource name=w58, byte count=u32 1000, error in (no error)=w57) -> (VISA resource name out=w54:refnum<visa-resource-name>, read buffer=w45:string, error out=w55:errorcluster)  [unwired: 1 out]
    n9 = Match Pattern(string=w45, regular expression="A") -> (before substring=w59:string)  [unwired: 1 in, 3 out]
    n10 = Concatenate Strings(w53, w45) -> (w52:string)
    n11 = property class="Instr" props=["Bytes at Port"](reference=w54, error in=w55) -> (error out=w44:errorcluster)  [unwired: 2 out]
    n12 = call <vilib>:"Sine Waveform.vi"("phase"=0.0, "amplitude"=220.0, "frequency"="Frequence Reseau") -> ("signal out"=w38:waveform(dbl))  [unwired: 7 in, 1 out]
    n13 = Decimal String To Number(string=w59) -> (number=w32:i32)  [unwired: 2 in, 1 out]
    "Amplitude ECG\n    Amplifiée" <- w32
    n14 = call <vilib>:"AC & DC Estimator PtByPt.vi"("signal"=w32) -> ("AC estimate (Vrms)"=w39:dbl)  [unwired: 2 in, 2 out]
    n15 = Subtract(x=w32, y=w39) -> (x-y=w37:dbl)
    n16 = Add(x=w38, y=w37) -> (x+y=w36:waveform(dbl))
    "Signal bruité" <- w36
    n17 = Greater?(x=w32, y=139) -> (0:w30:bool)
    "?" <- w30
    n18 = Unbundle By Name(w44) -> ("status"=w51:bool)
    n19 = case shown="True" w30 {
      frame False {
      }
      frame True {
        n20 = call <vilib>:"Beep.vi"("use system alert? (T)"=FALSE, "duration (msec)"=u32 100, "frequency (Hz)"=u32 1200) -> ()  [unwired: 9 in]
      }
    }
    n21 = Compound Arithmetic op=OR(w51, "?") -> (w49:bool)
    n22 = case shown="True" w49 {
      frame False {
      }
      frame True {
        n23 = call <vilib>:"Beep.vi"("use system alert? (T)"=FALSE, "duration (msec)"=u32 700, "frequency (Hz)"=u32 737) -> ()  [unwired: 9 in]
      }
    }
    n24 = call "Filter"("Lower Cut-Off"="Frequence de coupure", "Signal"=w36) -> ("Filtered Signal"=w33:dynamicdata)  [unwired: 8 in, 1 out]
    "Signal filtré" <- w33
    n25 = call "Build Table"("Enable"="ON/OFF", "Reset"="Reset", "Signals"=w32) -> ("Table"=→"Table 2":string[][])  [unwired: 7 in, 1 out]
    n26 = xnode "Spectral  2"("Signals"=w33) -> ("FFT - (Peak)"=→"FFT Signal filtré":dynamicdata)  [unwired: 1 in, 2 out]
    n27 = xnode "Spectral"("Signals"=w36) -> ("FFT - (Peak)"=→"FFT Signal bruité":cluster{"f0":dbl, "df":dbl, "magnitude":dbl[]})  [unwired: 1 in, 2 out]
  }
  n28 = VISA Discard Events(8:w15, 11:w14) -> (0:w16:errorcluster, 3:w17:refnum<visa-resource-name>)  [unwired: 2 in]
  n29 = VISA Close(VISA resource name=w17, error in (no error)=w16) -> ()  [unwired: 1 out]
